vi "运维调试_总磷总氮.vi"() -> ()   [LabVIEW 2016, in "斯坦道总磷总氮.lvlib"]
uses:
  <vilib>/Utility/miscctls.llb/LVPointTypeDef.ctl
  <vilib>/Utility/config.llb/NI_LVConfig.lvlib
  <vilib>/ptbypt/NI_PtbyPt.lvlib
panel:
  in  "总磷参数设置":bool
  in  "总氮参数设置":bool
  in  "模块启用":bool
  in  "串口设置":bool
  in  "备用系数一键写入":bool
  in  "公式一键写入":bool
  in  "流程路径":path=path "C:/Users/std/Documents/斯坦道流程文件/流程.xml"
  in  "曲线模型":cluster{"X^2":dbl, "X":dbl, "B":dbl}(xcontrol)
  out "字符串 2":string
  in  "质控参数设置":bool
  in  "总氮自动测试量程配置":T1
  in  "总磷自动测试量程配置":T1
  out "温度2":sgl
  out "温度1":sgl
  out "ADC":sgl
  out "固件版本号":string
  in  "数组":string[](array[string])
  in  "备用系数写入":bool
  in  "备用系数读取":bool
  in  "备用系数":T2
  in  "量程切换阈值写入":bool
  in  "量程切换阈值读取":bool
  in  "量程切换阈值":cluster{"阈值":dbl, "标液浓度":dbl}
  in  "参数下拉列表":enum16{"总磷", "总氮"}(ring)
  in  "量程下拉列表":enum16{"低量程", "高量程"}(ring)
  in  "测量模式下拉列表":enum16{"水样测量", "零点核查", "跨度核查", "标样核查", "加标回收"}(ring)
  in  "公式":cluster{"X^2":dbl, "X":dbl, "b":dbl}
  in  "写公式":bool
  in  "读公式":bool
  in  "返回":bool
  in  "设置":bool
  out "序列号":string="序列号"
  out "总氮测量数据":T3(xcontrol)
  out "总磷测量数据":T3(xcontrol)
  out "集成报警信息":string
  out "定时启动":bool
  out "总磷总氮运行状态":T4(xcontrol)
  in  "停止":bool
  in  "手动启动":bool
  in  "单步测试":bool
  in  "总磷氨氮调试":u16[](xcontrol)
  out "F3":sgl format="%#.6f"
  out "F2":sgl format="%#.6f"
  out "F1":sgl format="%#.6f"
  out "F0":sgl format="%#.6f"
  out "多列列表框":i32(listbox)
  # "参数设置"
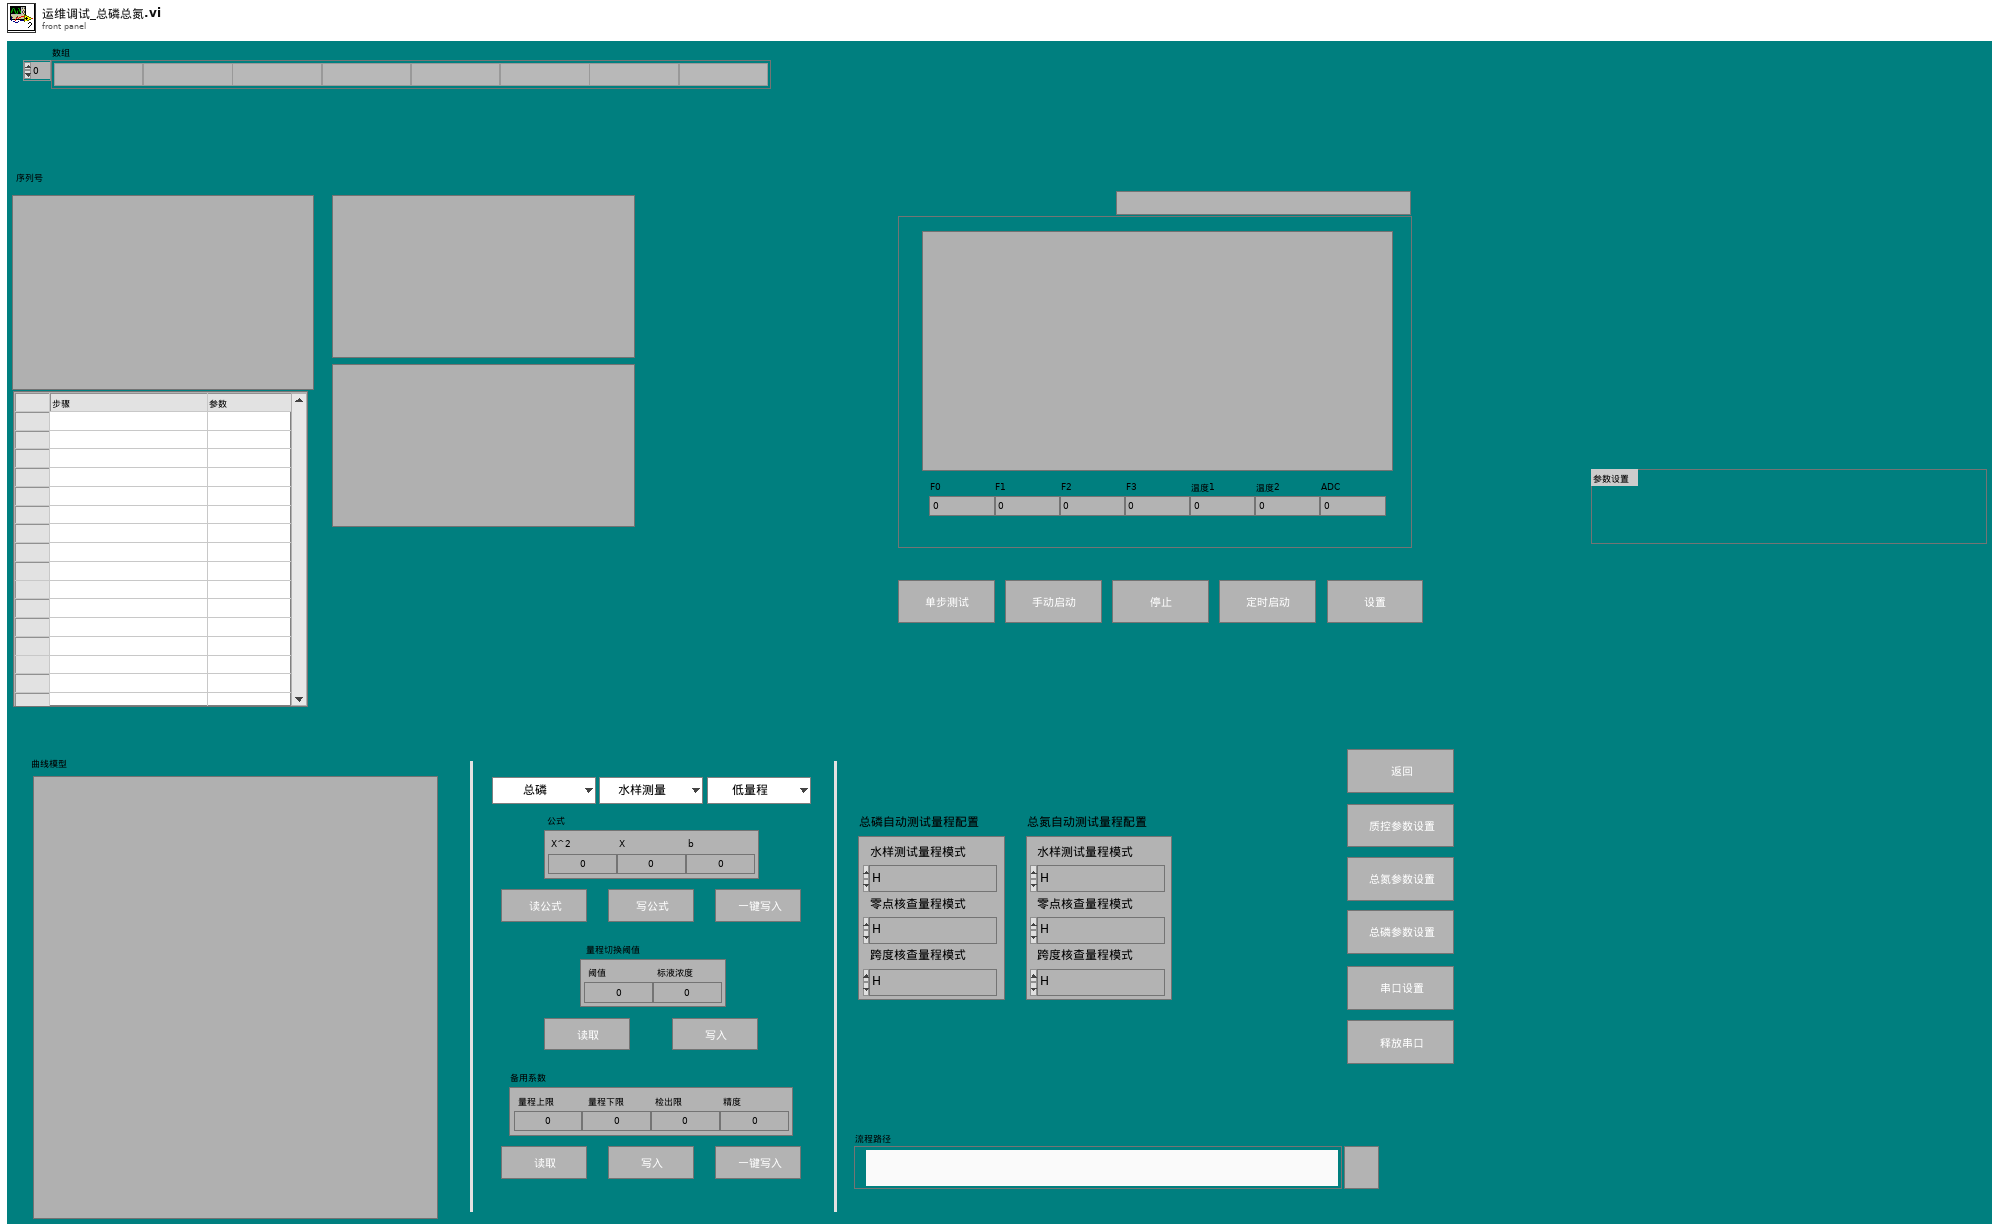
[diagram p1: front panel]
types:
  T1 = cluster{"水样测试量程模式":enum16{"H", "L", "AUTO"}, "空白核查量程模式":enum16{"H", "L", "AUTO"}, "跨度核查量程模式":enum16{"H", "L", "AUTO"}}
  T2 = cluster{"量程上限":dbl, "量程下限":dbl, "检出限":dbl, "精度":dbl}
  T3 = cluster{"flowid":u16, "测量精度":u16, "测量数据区":cluster{"因子编码":u32, "单位":u16, "标样参考值":sgl, "水样数据时间":timestamp, "水样实测值":sgl, "水样数据标识":string, "标样数据时间":timestamp, "标样实测值":sgl, "标样数据标识":string, "空白数据时间":timestamp, "空白实测值":sgl, "空白数据标识":string, "零点核查数据时间":timestamp, "零点核查实测值":sgl, "零点核查数据标识":string, "跨度核查数据时间":timestamp, "跨度核查实测值":sgl, "跨度核查数据标识":string, "加标回收数据时间":timestamp, "加标回收实测值":sgl, "加标回收数据标识":string, "平行样数据时间":timestamp, "平行样实测值":sgl, "平行样数据标识":string, "F0":sgl, "F1":sgl, "F2":sgl, "F3":sgl, "F4":sgl, "F5":sgl, "F6":sgl, "F7":sgl, "温度":sgl, "湿度":sgl, "X值":sgl}}
  T4 = cluster{"系统时间":timestamp, "工作状态":enum16{"空闲", "水样测试", "标样核查", "零点核查", "跨度核查", "空白测试", "平行样测试", "加标回收", "空白校准", "标样校准", "初始化（清洗）"}, "测量模式":enum16{"待机", "连续模式", "周期模式", "定点模式", "受控模式", "手动模式"}, "告警代码":u16, "故障代码":u16, "日志代码":u16, "软件版本":u16, "F0":sgl, "F1":sgl, "F2":sgl, "F3":sgl, "T":sgl, "H":sgl, "id":u16, "flowid":u16, "量程":u16, "总磷控温温度1":sgl, "营养盐控温温度2":sgl, "ADC":sgl}
  T5 = enum16{"启动测量", "标样核查", "零点核查", "跨度核查", "空白测试", "平行样测试", "加标回收", "空白校准", "标样校准", "初始化（清洗）", "停止测试", "仪器重启", "校时", "模式设置", "测量间隔设置"}
  T6 = cluster{"仪器测试类型":enum16{"启动测量", "标样核查", "零点核查", "跨度核查", "空白测试", "平行样测试", "加标回收", "空白校准", "标样校准", "初始化（清洗）", "停止测试", "仪器重启", "校时", "模式设置", "测量间隔设置"}, "周期设置类型":enum16{"定点启动", "间隔启动"}, "定时功能启用":bool, "定时间隔":dbl, "24H周期设置":bool[], "零点核查时间":u16, "跨度核查时间":u16, "质控频次":enum16{"关闭", "每天", "星期一", "星期二", "星期三", "星期四", "星期五", "星期六", "星期日"}}
  T7 = enum16{"关闭", "每天", "星期一", "星期二", "星期三", "星期四", "星期五", "星期六", "星期日"}
  T8 = enum32{"Bad", "Idle", "Run top level", "Running"}
  T9 = typedef "LVDateTimeRec.ctl" = cluster{"秒数的小数部分":dbl, "秒":i32, "分":i32, "时":i32, "日":i32, "月":i32, "年":i32, "天数（周）":i32, "天数（年）":i32, "DST":i32}
  T10 = typedef "LVPointTypeDef.ctl" = cluster{"Horizontal":i16, "Vertical":i16}
  T11 = cluster{"因子编码":u32, "单位":u16, "标样参考值":sgl, "水样数据时间":timestamp, "水样实测值":sgl, "水样数据标识":string, "标样数据时间":timestamp, "标样实测值":sgl, "标样数据标识":string, "空白数据时间":timestamp, "空白实测值":sgl, "空白数据标识":string, "零点核查数据时间":timestamp, "零点核查实测值":sgl, "零点核查数据标识":string, "跨度核查数据时间":timestamp, "跨度核查实测值":sgl, "跨度核查数据标识":string, "加标回收数据时间":timestamp, "加标回收实测值":sgl, "加标回收数据标识":string, "平行样数据时间":timestamp, "平行样实测值":sgl, "平行样数据标识":string, "F0":sgl, "F1":sgl, "F2":sgl, "F3":sgl, "F4":sgl, "F5":sgl, "F6":sgl, "F7":sgl, "温度":sgl, "湿度":sgl, "X值":sgl}
  T12 = enum16{"空闲", "水样测试", "标样核查", "零点核查", "跨度核查", "空白测试", "平行样测试", "加标回收", "空白校准", "标样校准", "初始化（清洗）"}
  T13 = typedef "NI_LVConfig.lvlib/Config Data RefNum.ctl" = refnum<k1>
  T14 = cluster{"启动模式":enum16{"跨度核查", "水样测量", "空白核查", "标样核查", "加标回收"}, "启动参数":u16, "量程":enum16{"低量程", "高量程"}}
  T15 = cluster{"时间标识":timestamp, "设备":string, "日志信息":string, "流程参数":string}
  T16 = cluster{"时间标识":timestamp, "设备":string, "日志信息":string}
  T17 = typedef "LVRowAndColumnUnsignedTypeDef.ctl" = cluster{"Row":u32, "Column":u32}
  T18 = cluster{"参数下拉列表":enum16{"总磷", "总氮"}, "测量模式下拉列表":enum16{"水样测量", "零点核查", "跨度核查", "标样核查", "加标回收"}, "量程下拉列表":enum16{"低量程", "高量程"}}
  T19 = cluster{"站号":u16, "量程切换":enum32{"H", "L", "AUTO"}, "控制命令":enum16{"启动测量", "标样核查", "零点核查", "跨度核查", "空白测试", "平行样测试", "加标回收", "空白校准", "标样校准", "初始化（清洗）", "停止测试", "仪器重启", "校时", "模式设置", "测量间隔设置"}, "模式设置":enum16{"待机", "连续模式", "周期模式", "定点模式", "受控模式", "手动模式"}, "测量间隔":u16}
  T20 = cluster{"总磷跨度值":dbl, "总磷零点标准液浓度":dbl, "总磷跨度标准液浓度":dbl, "总磷标准液标准浓度":dbl, "总氮跨度值":dbl, "总氮零点标准液浓度":dbl, "总氮跨度标准液浓度":dbl, "总氮标准液标准浓度":dbl}
  T21 = cluster{"确定":bool, "总磷跨度值":dbl, "总磷零点标准液浓度":dbl, "总磷跨度标准液浓度":dbl, "总磷标准液标准浓度":dbl, "总氮跨度值":dbl, "总氮零点标准液浓度":dbl, "总氮跨度标准液浓度":dbl, "总氮标准液标准浓度":dbl}
  T22 = cluster{"测量量程":dbl, "测量精度":dbl, "测量间隔":dbl, "消解温度":dbl, "消解时长":dbl, "空白校准时间":timestamp, "曲线截距":dbl, "曲线斜率":dbl, "测量检出限":dbl, "测量信号值":dbl, "线性相关系数":dbl, "二次多项式系数":dbl, "标样校准时间":timestamp, "稀释倍数":dbl, "三项式系数":dbl, "空白标定系数":dbl, "量程系数":dbl, "F0/ORPA":dbl, "F1/ORPB":dbl, "F2/ORPK":dbl, "F3":dbl, "F4":dbl, "F5":dbl, "F6":dbl, "F7":dbl, "X0/滴定数":dbl, "量程":dbl}
  T23 = cluster{"确定":bool, "测量量程":dbl, "测量精度":dbl, "测量间隔":dbl, "消解温度":dbl, "消解时长":dbl, "空白校准时间":timestamp, "曲线截距":dbl, "曲线斜率":dbl, "测量检出限":dbl, "测量信号值":dbl, "线性相关系数":dbl, "二次多项式系数":dbl, "标样校准时间":timestamp, "稀释倍数":dbl, "三项式系数":dbl, "空白标定系数":dbl, "量程系数":dbl, "F0/ORPA":dbl, "F1/ORPB":dbl, "F2/ORPK":dbl, "F3":dbl, "F4":dbl, "F5":dbl, "F6":dbl, "F7":dbl, "X0/滴定数":dbl, "量程":dbl}
  T24 = cluster{"控制命令":enum16{"启动测量", "标样核查", "零点核查", "跨度核查", "空白测试", "平行样测试", "加标回收", "空白校准", "标样校准", "初始化（清洗）", "停止测试", "仪器重启", "校时", "模式设置", "测量间隔设置"}, "周期设置类型":enum16{"定点启动", "间隔启动"}, "定时功能启用":bool, "定时间隔":dbl, "24H周期设置":bool[], "空白核查时间":u16, "跨度核查时间":u16, "质控频次":enum16{"关闭", "每天", "星期一", "星期二", "星期三", "星期四", "星期五", "星期六", "星期日"}}
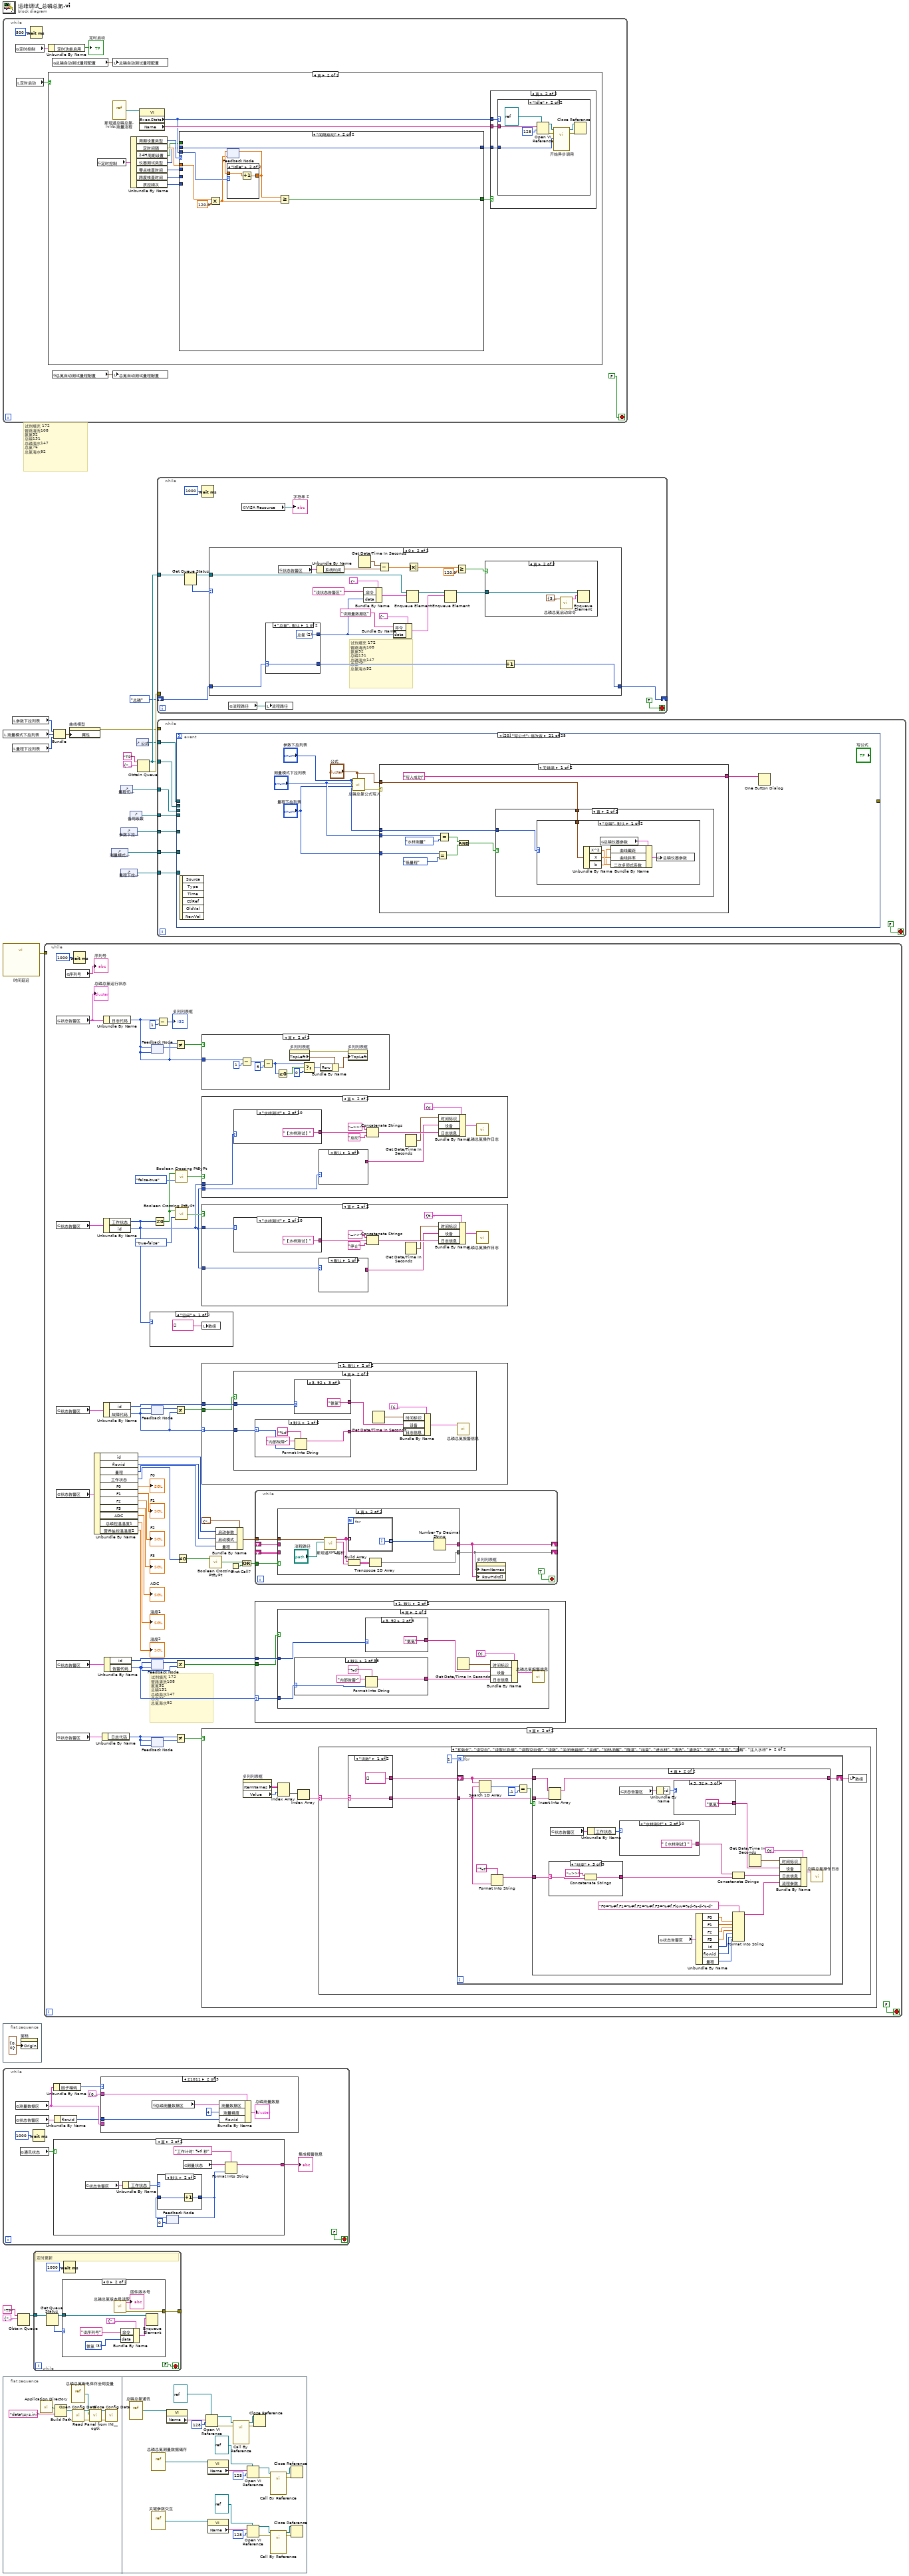
[diagram p0: block diagram]
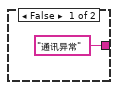
[diagram p3: hidden frame]
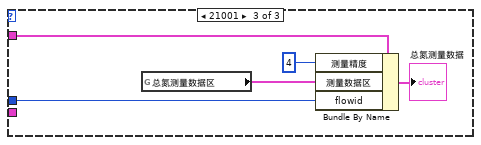
[diagram p6: hidden frame]
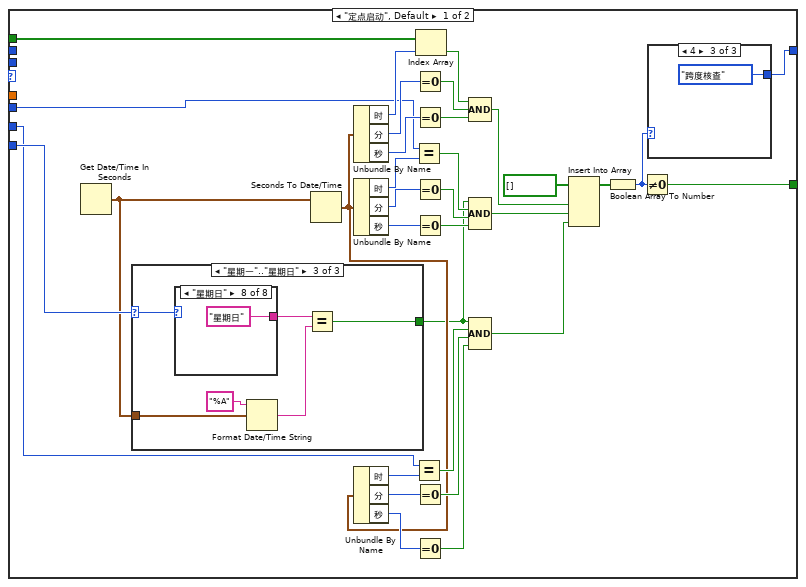
[diagram p8: hidden frame]
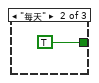
[diagram p10: hidden frame]
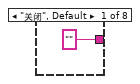
[diagram p11: hidden frame]
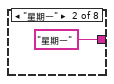
[diagram p12: hidden frame]
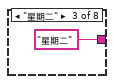
[diagram p13: hidden frame]
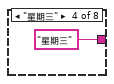
[diagram p14: hidden frame]
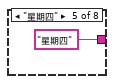
[diagram p15: hidden frame]
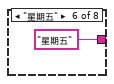
[diagram p16: hidden frame]
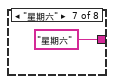
[diagram p17: hidden frame]
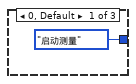
[diagram p18: hidden frame]
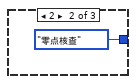
[diagram p19: hidden frame]
diagram:
  # "试剂填充 172 \n管路清洗108\n氨氮92\n总磷131\n总磷海水147\n总氮76\n总氮海水92"
  n1 = while {
    stop <- FALSE stop-if-true
    n2 = global read "总磷总氮断电保存全局变量.vi" "定时控制"() -> (w22:T6)
    n3 = local read "定时启动"() -> (w25:bool)
    n4 = Wait (ms)(milliseconds to wait=u32 500 ("等待时间（毫秒）")) -> ()  [unwired: 1 out]
    n5 = Unbundle By Name(w22) -> ("定时功能启用"=→"定时启动":bool)
    n6 = case shown="真" w25 {
      frame False {
      }
      frame True {
        n7 = global read "总磷总氮断电保存全局变量.vi" "定时控制"() -> (w40:T6)
        n8 = vi-ref "斯坦道总磷总氮.lvlib:测量流程.vi"() -> (w39:refnum<vi>)
        n9 = Unbundle By Name(w40) -> ("周期设置类型"=w37:enum16{"定点启动", "间隔启动"}, "定时间隔"=w35:dbl, "24H周期设置"=w34:bool[], "仪器测试类型"=w33:T5, "零点核查时间"=w32:u16, "跨度核查时间"=w31:u16, "质控频次"=w30:T7)
        n10 = property class="VI"(reference=w39) -> ("Exec.State"=w36:T8, "Name"=w38:string)  [unwired: 1 in, 2 out]
        n11 = case shown="\"间隔启动\"" w37 {
          tunnel: w35 -> [_ w96]
          tunnel: w34 -> [w64 _]
          tunnel: w36 -> [_ w99]
          tunnel: [w42 w94] -> w28
          tunnel: w33 -> [_ w92]
          tunnel: [w68 w92] -> w29
          tunnel: w30 -> [w67 _]
          tunnel: w32 -> [w60 _]
          tunnel: w31 -> [w49 _]
          frame "定点启动", Default {
            n12 = Get Date/Time In Seconds() -> (seconds since 1Jan1904=w66:timestamp)
            n13 = case shown="\"星期一\"..\"星期日\"" w67 {
              selector: w67 -> [_ _ w78]
              tunnel: w66 -> [_ _ w79]
              tunnel: [_ TRUE w75] -> w48
              frame "关闭", Default {
              }
              frame "每天" {
              }
              frame "星期一".."星期日" {
                n14 = case shown="\"星期日\"" w78 {
                  tunnel: ["" ("时间格式字符串(%c)") "星期一" ("时间格式字符串(%c)") "星期二" ("时间格式字符串(%c)") "星期三" ("时间格式字符串(%c)") "星期四" ("时间格式字符串(%c)") "星期五" ("时间格式字符串(%c)") "星期六" ("时间格式字符串(%c)") "星期日" ("时间格式字符串(%c)")] -> w77
                  frame "关闭", Default {
                  }
                  frame "星期一" {
                  }
                  frame "星期二" {
                  }
                  frame "星期三" {
                  }
                  frame "星期四" {
                  }
                  frame "星期五" {
                  }
                  frame "星期六" {
                  }
                  frame "星期日" {
                  }
                }
                n15 = Format Date/Time String(time format string (%c)="%A" ("时间格式字符串(%c)"), seconds (now)=w79) -> (date/time string=w76:string)  [unwired: 1 in]
                n16 = Equal?(x=w77, y=w76) -> (x = y?=w75:bool)
              }
            }
            n17 = Seconds To Date/Time(time stamp (now)=w66) -> (date time rec=w50:T9)  [unwired: 1 in]
            n18 = Unbundle By Name(w50) -> ("时"=w73:i32, "分"=w71:i32, "秒"=w72:i32)
            n19 = Unbundle By Name(w50) -> ("时"=w61:i32, "分"=w63:i32, "秒"=w62:i32)
            n20 = Unbundle By Name(w50) -> ("时"=w53:i32, "分"=w51:i32, "秒"=w52:i32)
            n21 = Equal?(x=w60, y=w61) -> (x = y?=w59:bool)
            n22 = Equal?(x=w49, y=w53) -> (x = y?=w54:bool)
            n23 = Equal To 0?(x=w71) -> (x = 0?=w70:bool)
            n24 = Equal To 0?(x=w72) -> (x = 0?=w69:bool)
            n25 = Equal To 0?(x=w63) -> (x = 0?=w58:bool)
            n26 = Equal To 0?(x=w62) -> (x = 0?=w57:bool)
            n27 = Equal To 0?(x=w51) -> (x = 0?=w55:bool)
            n28 = Equal To 0?(x=w52) -> (x = 0?=w56:bool)
            n29 = Index Array(array=w64, index=w73) -> (element=w65:bool)
            n30 = Compound Arithmetic op=AND ("复合运算")(w65, w70, w69) -> (w46:bool)
            n31 = Compound Arithmetic op=AND ("复合运算")(w48, w59, w58, w57) -> (w45:bool)
            n32 = Compound Arithmetic op=AND ("复合运算")(w48, w54, w55, w56) -> (w44:bool)
            n33 = Insert Into Array(array=bool[] [], new element #1=w46, new element #2=w45, new element #3=w44) -> (w43:bool[])  [unwired: 1 in]
            n34 = Boolean Array To Number(Boolean array=w43) -> (number=w41:u32)
            n35 = Not Equal To 0?(x=w41) -> (x != 0?=w42:bool)
            n36 = case shown="4" w41 {
              tunnel: [T5."启动测量" ("控制命令") T5."零点核查" ("控制命令") T5."跨度核查" ("控制命令")] -> w68
              frame 0, Default {
              }
              frame 2 {
              }
              frame 4 {
              }
            }
          }
          frame "间隔启动" {
            n37 = Multiply(x=w96, y=120.0) -> (x*y=w93:dbl)
            n38 = feedback #1(w93) -> (w98:dbl)
            n39 = case shown="\"Idle\"" w99 {
              tunnel: w98 -> [_ w101]
              tunnel: [_ w100] -> w97
              frame "Bad", Default {
              }
              frame "Idle" {
                n40 = Increment(x=w101) -> (x+1=w100:dbl)
              }
            }
            n41 = feedback-in #1(w97) -> ()
            n42 = Greater Or Equal?(x=w97, y=w93) -> (x >= y?=w94:bool)
          }
        }
        n43 = case shown="真" w28 {
          tunnel: w38 -> [_ w104]
          tunnel: w29 -> [_ w103]
          tunnel: w36 -> [_ w102]
          frame False {
          }
          frame True {
            n44 = case shown="\"Idle\"" w102 {
              tunnel: w104 -> [_ w108]
              tunnel: w103 -> [_ w105]
              frame "Bad", Default {
              }
              frame "Idle" {
                n45 = Open VI Reference(type specifier VI Refnum (for type only)=refnum<vi> refnum, vi path=w108, options=128 ("选项")) -> (vi reference=w109:refnum<vi>, error out=w110:errorcluster)  [unwired: 3 in]
                n46 = call-by-ref "开始异步调用"(reference=w109, error in=w110, "控制命令"=w105) -> (reference out=w111:refnum<vi>, error out=w112:errorcluster)  [unwired: 11 in]
                n47 = Close Reference(reference=w111, error in (no error)=w112) -> ()  [unwired: 1 out]
              }
            }
          }
        }
      }
    }
    n48 = global read "总磷总氮断电保存全局变量.vi" "总磷自动测试量程配置"() -> (w23:T1)
    n49 = global read "总磷总氮断电保存全局变量.vi" "总氮自动测试量程配置"() -> (w24:T1)
    n50 = local write "总磷自动测试量程配置"(w23) -> ()
    n51 = local write "总氮自动测试量程配置"(w24) -> ()
  }
  n52 = local read "测量模式下拉列表"() -> (w3:enum16{"水样测量", "零点核查", "跨度核查", "标样核查", "加标回收"})
  n53 = call "时间延迟"() -> ("error out"=w9:errorcluster)  [unwired: 11 in]
  n54 = flat-sequence {
    frame #0 {
      n55 = property on="窗格" class="Pane"("Origin"=T10 {"Horizontal"=0, "Vertical"=0} ("原点")) -> ()  [unwired: 2 in, 2 out]
    }
  }
  n56 = while {
    stop <- FALSE stop-if-true
    n57 = global read "VAR总磷总氮全局变量.vi" "测量数据区"() -> (w120:T11)
    n58 = global read "VAR总磷总氮全局变量.vi" "状态告警区"() -> (w116:T4)
    n59 = global read "VAR总磷总氮全局变量.vi" "通讯状态"() -> (w118:bool)
    n60 = Wait (ms)(milliseconds to wait=u32 1000 ("等待时间（毫秒）")) -> ()  [unwired: 1 out]
    n61 = Unbundle By Name(w120) -> ("因子编码"=w119:u32)
    n62 = case shown="真" w118 {
      tunnel: ["通讯异常" ("集成报警信息") w125] -> w117
      frame False {
      }
      frame True {
        n63 = global read "VAR总磷总氮全局变量.vi" "状态告警区"() -> (w131:T4)
        n64 = Unbundle By Name(w131) -> ("工作状态"=w130:T12)
        n65 = feedback #2(0) -> (w128:i32)
        n66 = case shown="默认" w130 {
          tunnel: w128 -> [_ w133]
          tunnel: [_ w132] -> w126
          frame "空闲" {
          }
          frame Default {
            n67 = Increment(x=w133) -> (x+1=w132:i32)
          }
        }
        n68 = feedback-in #2(w126) -> ()
        n69 = global read "VAR总磷总氮全局变量.vi" "测量状态"() -> (w124:string)
        n70 = Format Into String(format string="工作计时: %d 秒" ("格式字符串"), initial string=w124, w126) -> (resulting string=w125:string)  [unwired: 1 in, 1 out]
      }
    }
    "集成报警信息" <- w117
    n71 = Unbundle By Name(w116) -> ("flowid"=w115:u16)
    n72 = case shown="21011" w119 {
      tunnel: w120 -> [_ _ _]
      tunnel: w115 -> [_ w136 w142]
      tunnel: T3 {"flowid"=0, "测量精度"=0, "测量数据区"={"因子编码"=0, "单位"=0, "标样参考值"=0.0, "水样数据时间"=timestamp(0 s since 1904-01-01), "水样实测值"=0.0, "水样数据标识"="", "标样数据时间"=timestamp(0 s since 1904-01-01), "标样实测值"=0.0, "标样数据标识"="", "空白数据时间"=timestamp(0 s since 1904-01-01), "空白实测值"=0.0, "空白数据标识"="", "零点核查数据时间"=timestamp(0 s since 1904-01-01), "零点核查实测值"=0.0, "零点核查数据标识"="", "跨度核查数据时间"=timestamp(0 s since 1904-01-01), "跨度核查实测值"=0.0, "跨度核查数据标识"="", "加标回收数据时间"=timestamp(0 s since 1904-01-01), "加标回收实测值"=0.0, "加标回收数据标识"="", "平行样数据时间"=timestamp(0 s since 1904-01-01), "平行样实测值"=0.0, "平行样数据标识"="", "F0"=0.0, "F1"=0.0, "F2"=0.0, "F3"=0.0, "F4"=0.0, "F5"=0.0, "F6"=0.0, "F7"=0.0, "温度"=0.0, "湿度"=0.0, "X值"=0.0}} ("总氮测量数据") -> [_ w135 w141]
      frame Default {
      }
      frame 21011 {
        n73 = global read "VAR总磷总氮全局变量.vi" "总磷测量数据区"() -> (w134:T11)
        n74 = Bundle By Name(cluster=w135, "测量数据区"=w134, "测量精度"=u16 4, "flowid"=w136) -> (→"总磷测量数据":T3)
      }
      frame 21001 {
        n75 = global read "VAR总磷总氮全局变量.vi" "总氮测量数据区"() -> (w139:T11)
        n76 = Bundle By Name(cluster=w141, "测量精度"=u16 4, "测量数据区"=w139, "flowid"=w142) -> (→"总氮测量数据":T3)
      }
    }
  }
  n77 = flat-sequence {
    frame #0 {
      n78 = call <vilib>:"Application Directory.vi"() -> ("Application Directory"=w151:path)
      n79 = Build Path(base path=w151, name or relative path="data\\sys.ini" ("名称或相对路径")) -> (appended path=w149:path)
      n80 = vi-ref "总磷总氮断电保存全局变量.vi"() -> (w147:refnum<vi>)
      n81 = call <vilib>:"Open Config Data.vi"("configuration file path"=w149) -> ("error out"=w145:errorcluster, "refnum"=w148:T13)  [unwired: 8 in, 1 out]
      n82 = call <userlib>:"Read Panel from INI__ogtk.vi"("error in (no error)"=w145, "VI ref"=w147, "refnum"=w148) -> ("error out"=w144:errorcluster, "refnum out"=w146:T13)  [unwired: 7 in]
      n83 = call <vilib>:"Close Config Data.vi"("error in (no error)"=w144, "refnum"=w146) -> ()  [unwired: 8 in, 2 out]
    }
    frame #1 {
      n84 = vi-ref "总磷总氮通讯.vi"() -> (w175:refnum<vi>)
      n85 = vi-ref "总磷总氮测量数据储存.vi"() -> (w167:refnum<vi>)
      n86 = vi-ref "关键参数交互.vi"() -> (w152:refnum<vi>)
      n87 = property class="VI"(reference=w175) -> ("Name"=w174:string)  [unwired: 1 in, 2 out]
      n88 = Open VI Reference(type specifier VI Refnum (for type only)=refnum<vi> refnum, vi path=w174, options=128 ("选项")) -> (vi reference=w172:refnum<vi>, error out=w170:errorcluster)  [unwired: 3 in]
      n89 = property class="VI"(reference=w167) -> ("Name"=w160:string)  [unwired: 1 in, 2 out]
      n90 = property class="VI"(reference=w152) -> ("Name"=w159:string)  [unwired: 1 in, 2 out]
      n91 = call-by-ref "?"(reference=w172, error in=w170) -> (reference out=w168:refnum<vi>, error out=w169:errorcluster)  [unwired: 12 in]
      n92 = Open VI Reference(type specifier VI Refnum (for type only)=refnum<vi> refnum, vi path=w160, options=128 ("选项")) -> (vi reference=w162:refnum<vi>, error out=w164:errorcluster)  [unwired: 3 in]
      n93 = Open VI Reference(type specifier VI Refnum (for type only)=refnum<vi> refnum, vi path=w159, options=128 ("选项")) -> (vi reference=w157:refnum<vi>, error out=w155:errorcluster)  [unwired: 3 in]
      n94 = Close Reference(reference=w168, error in (no error)=w169) -> ()  [unwired: 1 out]
      n95 = call-by-ref "?"(reference=w162, error in=w164) -> (reference out=w166:refnum<vi>, error out=w165:errorcluster)  [unwired: 12 in]
      n96 = call-by-ref "?"(reference=w157, error in=w155) -> (reference out=w153:refnum<vi>, error out=w154:errorcluster)  [unwired: 12 in]
      n97 = Close Reference(reference=w166, error in (no error)=w165) -> ()  [unwired: 1 out]
      n98 = Close Reference(reference=w153, error in (no error)=w154) -> ()  [unwired: 1 out]
    }
  }
  n99 = local read "参数下拉列表"() -> (w2:enum16{"总磷", "总氮"})
  n100 = local read "量程下拉列表"() -> (w1:enum16{"低量程", "高量程"})
  n101 = Obtain Queue(name (unnamed)="TP" ("名称（未命名）"), element data type=cluster{"命令":string, "data":variant} {"命令"="", "data"=variant}) -> (queue out=w6:refnum<queue>)  [unwired: 3 in, 2 out]
  n102 = while {
    tunnel: w6 -> [w180]
    tunnel: [w178] -> _
    stop <- FALSE stop-if-true
    # "定时更新"
    n103 = Get Queue Status(queue=w180) -> (queue out=w177:refnum<queue>, # elements in queue=w176:i32)  [unwired: 2 in, 6 out]
    n104 = case shown="0" w176 {
      tunnel: w177 -> [_ w185]
      tunnel: [_ w182] -> w178
      frame Default {
      }
      frame 0 {
        w186 = u16 3 items=["总磷"=1, "氨氮"=3] ("站号")
        n105 = call "总磷总氮版本号读取.vi"() -> ("error out"=w182:errorcluster, "固件版本号"=→"固件版本号":string)  [unwired: 10 in]
        n106 = Bundle By Name(cluster=cluster{"命令":string, "data":variant} {"命令"="", "data"=variant} ("元素"), "命令"="读序列号", "data"=w186) -> (w184:cluster{"命令":string, "data":variant})
        n107 = Enqueue Element(queue=w185, element=w184) -> ()  [unwired: 2 in, 3 out]
      }
    }
    n108 = Wait (ms)(milliseconds to wait=u32 1000 ("等待时间（毫秒）")) -> ()  [unwired: 1 out]
  }
  n109 = while {
    tunnel: w9 -> [_]
    stop <- FALSE stop-if-true
    # "试剂填充 172 \n管路清洗108\n氨氮92\n总磷131\n总磷海水147\n总氮76\n总氮海水92"
    n110 = global read "VAR总磷总氮全局变量.vi" "状态告警区"() -> (w222:T4)
    "总磷总氮运行状态" <- w222
    n111 = global read "VAR总磷总氮全局变量.vi" "状态告警区"() -> (w209:T4)
    n112 = global read "VAR总磷总氮全局变量.vi" "状态告警区"() -> (w214:T4)
    n113 = global read "VAR总磷总氮全局变量.vi" "状态告警区"() -> (w230:T4)
    n114 = global read "VAR总磷总氮全局变量.vi" "状态告警区"() -> (w219:T4)
    n115 = global read "VAR总磷总氮全局变量.vi" "状态告警区"() -> (w207:T4)
    n116 = global read "VAR总磷总氮全局变量.vi" "序列号"() -> (→"序列号":string)
    n117 = Wait (ms)(milliseconds to wait=u32 1000 ("等待时间（毫秒）")) -> ()  [unwired: 1 out]
    n118 = Unbundle By Name(w230) -> ("id"=w227:u16, "flowid"=w229:u16, "量程"=w228:u16, "工作状态"=w197:T12, "F0"=→"F0":sgl, "F1"=→"F1":sgl, "F2"=→"F2":sgl, "F3"=→"F3":sgl, "ADC"=→"ADC":sgl, "总磷控温温度1"=→"温度1":sgl, "营养盐控温温度2"=→"温度2":sgl)
    n119 = Unbundle By Name(w207) -> ("日志代码"=w206:u16)
    n120 = Unbundle By Name(w222) -> ("日志代码"=w203:u16)
    n121 = Unbundle By Name(w209) -> ("工作状态"=w190:T12, "id"=w189:u16)
    n122 = Unbundle By Name(w214) -> ("id"=w213:u16, "故障代码"=w210:u16)
    n123 = Unbundle By Name(w219) -> ("id"=w218:u16, "告警代码"=w215:u16)
    n124 = case shown="\"空闲\"" w190 {
      frame "空闲" {
        n125 = local write "数组"(string[] [] ("数组")) -> ()
      }
      frame "水样测试", Default {
      }
    }
    n126 = feedback-in #3(w203) -> ()
    n127 = feedback #3(w203) -> (w235:u16)
    n128 = feedback #4(w210) -> (w211:u16)
    n129 = feedback-in #4(w210) -> ()
    n130 = feedback #5(w215) -> (w216:u16)
    n131 = feedback-in #5(w215) -> ()
    n132 = feedback #6(w206) -> (w208:u16)
    n133 = feedback-in #6(w206) -> ()
    n134 = Not Equal To 0?(x=w190) -> (x != 0?=w192:bool)
    n135 = Subtract(x=w203, y=1) -> (x-y=→"多列列表框":i32)
    n136 = Not Equal?(x=w203, y=w235) -> (x != y?=w234:bool)
    n137 = Not Equal?(x=w211, y=w210) -> (x != y?=w212:bool)
    n138 = Not Equal?(x=w216, y=w215) -> (x != y?=w217:bool)
    n139 = Not Equal?(x=w206, y=w208) -> (x != y?=w205:bool)
    n140 = call <vilib>:"Boolean Crossing PtByPt.vi"("direction"=enum16{"either", "false-true", "true-false"}."false-true", "input"=w192) -> ("crossing"=w194:bool)  [unwired: 1 in]
    n141 = call <vilib>:"Boolean Crossing PtByPt.vi"("direction"=enum16{"either", "false-true", "true-false"}."true-false", "input"=w192) -> ("crossing"=w191:bool)  [unwired: 1 in]
    n142 = Not Equal To 0?(x=w197) -> (x != 0?=w232:bool)
    n143 = case shown="真" w234 {
      tunnel: w203 -> [_ w445]
      frame False {
      }
      frame True {
        n144 = Subtract(x=w445, y=1) -> (x-y=w443:i32)
        n145 = Subtract(x=w443, y=5) -> (x-y=w447:i32)
        n146 = Greater Or Equal To 0?(x=w447) -> (x >= 0?=w446:bool)
        n147 = property on="多列列表框" class="MCListbox (严格)"() -> (error out=w451:errorcluster, "TopLeft"=w452:T17)  [unwired: 2 in, 1 out]
        n148 = Select(t=w447, s=w446, f=0) -> (s? t:f=w448:i32)
        n149 = Bundle By Name(cluster=w452, "Row"=w448) -> (w453:T17)
        n150 = property on="多列列表框" class="MCListbox (严格)"(error in=w451, "TopLeft"=w453) -> ()  [unwired: 1 in, 2 out]
      }
    }
    n151 = case shown="真" w194 {
      tunnel: w190 -> [_ w262]
      tunnel: w189 -> [_ w261]
      frame False {
      }
      frame True {
        n152 = case shown="\"水样测试\"" w262 {
          tunnel: [_ "【水样测试】" ("字符串") "【标样核查】" ("字符串") "【零点核查】" ("字符串") "【跨度核查】" ("字符串") "【空白测试】" ("字符串") "【平行样测试】" ("字符串") "【加标回收】" ("字符串") "【空白校准】" ("字符串") "【标样校准】" ("字符串")] -> w269
          frame "空闲", Default {
          }
          frame "水样测试" {
          }
          frame "标样核查" {
          }
          frame "零点核查" {
          }
          frame "跨度核查" {
          }
          frame "空白测试" {
          }
          frame "平行样测试" {
          }
          frame "加标回收" {
          }
          frame "空白校准" {
          }
          frame "标样校准" {
          }
        }
        n153 = case shown="默认" w261 {
          tunnel: [_ "总磷" ("table输入") "氨氮" ("table输入") "总氮" ("table输入")] -> w265
          frame Default {
          }
          frame 1, 131 {
          }
          frame 3, 92 {
          }
          frame 2, 76 {
          }
        }
        n154 = Concatenate Strings("-->>" ("字符串"), w269, "启动" ("字符串")) -> (w268:string)
        n155 = Get Date/Time In Seconds() -> (seconds since 1Jan1904=w266:timestamp)
        n156 = Bundle By Name(cluster=T15 {"时间标识"=timestamp(0 s since 1904-01-01), "设备"="", "日志信息"="", "流程参数"=""} ("data in"), "时间标识"=w266, "设备"=w265, "日志信息"=w268) -> (w260:T15)
        n157 = call "总磷总氮操作日志.vi"("data in"=w260) -> ()  [unwired: 11 in]
      }
    }
    n158 = case shown="真" w191 {
      tunnel: w190 -> [_ w240]
      tunnel: w189 -> [_ w239]
      frame False {
      }
      frame True {
        n159 = case shown="\"水样测试\"" w240 {
          tunnel: [_ "【水样测试】" ("字符串") "【标样核查】" ("字符串") "【零点核查】" ("字符串") "【跨度核查】" ("字符串") "【空白测试】" ("字符串") "【平行样测试】" ("字符串") "【加标回收】" ("字符串") "【空白校准】" ("字符串") "【标样校准】" ("字符串")] -> w247
          frame "空闲", Default {
          }
          frame "水样测试" {
          }
          frame "标样核查" {
          }
          frame "零点核查" {
          }
          frame "跨度核查" {
          }
          frame "空白测试" {
          }
          frame "平行样测试" {
          }
          frame "加标回收" {
          }
          frame "空白校准" {
          }
          frame "标样校准" {
          }
        }
        n160 = case shown="默认" w239 {
          tunnel: [_ "总磷" ("table输入") "氨氮" ("table输入") "总氮" ("table输入")] -> w243
          frame Default {
          }
          frame 1, 131 {
          }
          frame 3, 92 {
          }
          frame 2, 76 {
          }
        }
        n161 = Concatenate Strings("-->>" ("字符串"), w247, "停止" ("字符串")) -> (w246:string)
        n162 = Get Date/Time In Seconds() -> (seconds since 1Jan1904=w244:timestamp)
        n163 = Bundle By Name(cluster=T15 {"时间标识"=timestamp(0 s since 1904-01-01), "设备"="", "日志信息"="", "流程参数"=""} ("data in"), "时间标识"=w244, "设备"=w243, "日志信息"=w246) -> (w238:T15)
        n164 = call "总磷总氮操作日志.vi"("data in"=w238) -> ()  [unwired: 11 in]
      }
    }
    n165 = case shown="1, 默认" w210 {
      selector: w210 -> [_ w350]
      tunnel: w213 -> [_ w351]
      tunnel: w212 -> [_ w349]
      frame 0 {
      }
      frame 1, Default {
        n166 = case shown="真" w349 {
          tunnel: w351 -> [_ w358]
          tunnel: w350 -> [_ w353]
          frame False {
          }
          frame True {
            n167 = case shown="默认" w353 {
              selector: w353 -> [w360 _ _ _ _ _]
              tunnel: [w359 "无故障" "电机故障" "温度故障" "通讯故障" "滴定故障"] -> w352
              frame Default {
                n168 = Format Into String(format string="%d" ("格式字符串"), initial string="内部故障-" ("工作状态"), w360) -> (resulting string=w359:string)  [unwired: 1 in, 1 out]
              }
              frame 0 {
              }
              frame 1 {
              }
              frame 2 {
              }
              frame 3 {
              }
              frame 4 {
              }
            }
            n169 = case shown="3, 92" w358 {
              tunnel: [_ "总磷" ("table输入") "氨氮" ("table输入") "总氮" ("table输入")] -> w354
              frame Default {
              }
              frame 1, 131 {
              }
              frame 3, 92 {
              }
              frame 2, 76 {
              }
            }
            n170 = Get Date/Time In Seconds() -> (seconds since 1Jan1904=w355:timestamp)
            n171 = Bundle By Name(cluster=T16 {"时间标识"=timestamp(0 s since 1904-01-01), "设备"="", "日志信息"=""} ("data in"), "时间标识"=w355, "设备"=w354, "日志信息"=w352) -> (w356:T16)
            n172 = call "总磷总氮报警信息.vi"("data in"=w356) -> ()  [unwired: 10 in, 1 out]
          }
        }
      }
    }
    n173 = case shown="真" w205 {
      frame False {
      }
      frame True {
        n174 = property on="多列列表框" class="MCListbox (严格)"() -> ("ItemNames"=w285:string[][], "Value"=w286:i32)  [unwired: 2 in, 2 out]
        n175 = Index Array(array=w285, index (row)=w286) -> (element=w284:string[])  [unwired: 1 in]
        n176 = Index Array(array=w284) -> (element=w283:string)  [unwired: 1 in]
        n177 = case shown="\"初始化\", \"读空白\", \"读取比色值\", \"读取空白值\", \"读数\", \"关闭电磁阀\", \"关阀\", \"加热消解\", \"降温\", \"结束\", \"进水样\", \"清洗\", \"清洗1\", \"润洗\", \"显色\", \"消解\", \"注入水样\"" w283 {
          selector: w283 -> [_ w289]
          frame Default {
          }
          frame "初始化", "读空白", "读取比色值", "读取空白值", "读数", "关闭电磁阀", "关阀", "加热消解", "降温", "结束", "进水样", "清洗", "清洗1", "润洗", "显色", "消解", "注入水样" {
            n178 = case shown="\"读数\"" w289 {
              selector: w289 -> [w293 w295]
              tunnel: [w293 w295] -> w288
              tunnel: [string[] [] ("数组") "数组"] -> w287
              frame "读数" {
              }
              frame Default {
              }
            }
            n179 = for {
              N: 1 -> [_]
              tunnel: w288 -> [w297]
              shift-right: [w296] -> w290
              shift-left: w287 -> [w298]
              n180 = Search 1D Array(1D array=w298, element=w297) -> (index of element=w301:i32)  [unwired: 1 in]
              n181 = Format Into String(format string="%s" ("格式字符串"), w297) -> (resulting string=w302:string)  [unwired: 2 in, 1 out]
              n182 = Equal?(x=w301, y=-1) -> (x = y?=w299:bool)
              n183 = case shown="真" w299 {
                tunnel: w302 -> [_ w310]
                tunnel: w298 -> [w304 w314]
                tunnel: w297 -> [_ w313]
                tunnel: [w304 w312] -> w296
                frame False {
                }
                frame True {
                  n184 = Insert Into Array(array=w314, new element=w313) -> (w312:string[])  [unwired: 1 in]
                  n185 = case shown="\"结束\"" w310 {
                    selector: w310 -> [w339 w342 w345]
                    tunnel: [w339 w341 w344] -> w309
                    frame Default {
                    }
                    frame "初始化" {
                      n186 = Concatenate Strings("-->>" ("字符串"), w342) -> (w341:string)
                    }
                    frame "结束" {
                      n187 = Concatenate Strings("-->>" ("字符串"), w345) -> (w344:string)
                    }
                  }
                  n188 = global read "VAR总磷总氮全局变量.vi" "状态告警区"() -> (w308:T4)
                  n189 = Unbundle By Name(w308) -> ("工作状态"=w307:T12)
                  n190 = global read "VAR总磷总氮全局变量.vi" "状态告警区"() -> (w329:T4)
                  n191 = case shown="\"水样测试\"" w307 {
                    tunnel: [_ "【水样测试】" ("字符串") "【标样核查】" ("字符串") "【零点核查】" ("字符串") "【跨度核查】" ("字符串") "【空白测试】" ("字符串") "【平行样测试】" ("字符串") "【加标回收】" ("字符串") "【空白校准】" ("字符串") "【标样校准】" ("字符串")] -> w305
                    frame "空闲", Default {
                    }
                    frame "水样测试" {
                    }
                    frame "标样核查" {
                    }
                    frame "零点核查" {
                    }
                    frame "跨度核查" {
                    }
                    frame "空白测试" {
                    }
                    frame "平行样测试" {
                    }
                    frame "加标回收" {
                    }
                    frame "空白校准" {
                    }
                    frame "标样校准" {
                    }
                  }
                  n192 = Unbundle By Name(w329) -> ("id"=w328:u16)
                  n193 = global read "VAR总磷总氮全局变量.vi" "状态告警区"() -> (w324:T4)
                  n194 = case shown="3, 92" w328 {
                    tunnel: [_ "总磷" ("table输入") "氨氮" ("table输入") "总氮" ("table输入")] -> w326
                    frame Default {
                    }
                    frame 1, 131 {
                    }
                    frame 3, 92 {
                    }
                    frame 2, 76 {
                    }
                  }
                  n195 = Unbundle By Name(w324) -> ("F0"=w321:sgl, "F1"=w320:sgl, "F2"=w319:sgl, "F3"=w318:sgl, "id"=w317:u16, "flowid"=w316:u16, "量程"=w315:u16)
                  n196 = Concatenate Strings(w305, w309) -> (w306:string)
                  n197 = Format Into String(format string="F0=%#f,F1=%#f,F2=%#f,F3=%#f,Flow=%d-%-d-%-d" ("格式字符串"), w321, w320, w319, w318, w317, w316, w315) -> (resulting string=w322:string)  [unwired: 2 in, 1 out]
                  n198 = Get Date/Time In Seconds() -> (seconds since 1Jan1904=w325:timestamp)
                  n199 = Bundle By Name(cluster=T15 {"时间标识"=timestamp(0 s since 1904-01-01), "设备"="", "日志信息"="", "流程参数"=""} ("data in"), "时间标识"=w325, "设备"=w326, "日志信息"=w306, "流程参数"=w322) -> (w327:T15)
                  n200 = call "总磷总氮操作日志.vi"("data in"=w327) -> ()  [unwired: 11 in]
                }
              }
            }
            n201 = local write "数组"(w290) -> ()
          }
        }
      }
    }
    n202 = call <vilib>:"Boolean Crossing PtByPt.vi"("input"=w232) -> ("crossing"=w196:bool)  [unwired: 2 in]
    n203 = Bundle By Name(cluster=T14 {"启动模式"=enum."跨度核查", "启动参数"=1, "量程"=enum."低量程"} ("参数簇"), "启动参数"=w227, "启动模式"=w229, "量程"=w228) -> (w221:T14)
    n204 = First Call?() -> (First Call?: T/F=w233:bool)
    n205 = Or(x=w196, y=w233) -> (x .or. y?=w231:bool)
    n206 = while {
      tunnel: w231 -> [w431]
      tunnel: w221 -> [w430]
      shift-right: [w425] -> _
      shift-left: _ -> [w427]
      shift-right: [w426] -> _
      shift-left: _ -> [w428]
      stop <- TRUE stop-if-true
      n207 = case shown="真" w431 {
        tunnel: [w433 w441] -> w426
        tunnel: [w432 w440] -> w425
        tunnel: w430 -> [_ w435]
        tunnel: w428 -> [w433 _]
        tunnel: w427 -> [w432 _]
        frame False {
        }
        frame True {
          n208 = call "斯坦道XML解析.vi"("添加的路径"="流程路径", "参数簇"=w435) -> ("步骤时间"=w436:string[], "步骤名"=w438:string[])  [unwired: 8 in]
          n209 = for {
            tunnel: w438 -> [_] mode=indexing
            tunnel: [w442] -> w439 mode=indexing
            i -> [w442]
          }
          n210 = Build Array(w438, w436) -> (w437:string[][])
          n211 = Transpose 2D Array(2D array=w437) -> (transposed array=w440:string[][])
          n212 = Number To Decimal String(number=w439) -> (decimal integer string=w441:string[])  [unwired: 1 in]
        }
      }
      n213 = property on="多列列表框" class="MCListbox (严格)"("ItemNames"=w425, "RowHdrs[]"=w426) -> ()  [unwired: 2 in, 2 out]
    }
    n214 = case shown="1, 默认" w215 {
      selector: w215 -> [_ w372]
      tunnel: w218 -> [_ w373]
      tunnel: w217 -> [_ w371]
      frame 0 {
      }
      frame 1, Default {
        n215 = case shown="真" w371 {
          tunnel: w373 -> [_ w380]
          tunnel: w372 -> [_ w374]
          frame False {
          }
          frame True {
            n216 = case shown="默认" w374 {
              selector: w374 -> [w382 _ _ _ _ _ _ _ _ _ _ _ _ _ _ _ _ _ _ _ _ _ _ _ _ _ _ _ _ _ _ _ _ _ _ _ _ _]
              tunnel: [w381 "无告警" "缺试剂告警" "缺水样告警" "缺蒸馏水告警" "缺标液告警" "仪表漏液告警" "标定异常告警" "超量程告警" "加热异常" "低试剂预警" "超上限告警" "超下限告警" "仪表内部其他异常" "滴定异常告警" "电极异常告警" "量程切换告警" "参数设置告警" "PH电极电位异常" "电导率电极异常" "浊度光度异常" "溶解氧电极异常" "溶解氧光强异常" "温度异常告警" "PH异常告警" "溶解氧异常告警" "电导率异常告警" "浊度异常告警" "叶绿素异常告警" "藻密度异常告警" "蓝绿藻异常告警" "ORP异常告警" "氨氮异常告警" "清洁刷异常告警" "SD卡异常告警" "蓝牙异常告警" "WiFi异常告警" "流程异常告警"] -> w375
              frame Default {
                n217 = Format Into String(format string="%d" ("格式字符串"), initial string="内部告警-" ("工作状态"), w382) -> (resulting string=w381:string)  [unwired: 1 in, 1 out]
              }
              frame 0 {
              }
              frame 1 {
              }
              frame 2 {
              }
              frame 3 {
              }
              frame 4 {
              }
              frame 5 {
              }
              frame 6 {
              }
              frame 7 {
              }
              frame 8 {
              }
              frame 9 {
              }
              frame 10 {
              }
              frame 11 {
              }
              frame 12 {
              }
              frame 13 {
              }
              frame 14 {
              }
              frame 15 {
              }
              frame 16 {
              }
              frame 17 {
              }
              frame 18 {
              }
              frame 19 {
              }
              frame 20 {
              }
              frame 21 {
              }
              frame 22 {
              }
              frame 23 {
              }
              frame 24 {
              }
              frame 25 {
              }
              frame 26 {
              }
              frame 27 {
              }
              frame 28 {
              }
              frame 29 {
              }
              frame 30 {
              }
              frame 31 {
              }
              frame 32 {
              }
              frame 33 {
              }
              frame 34 {
              }
              frame 35 {
              }
              frame 36 {
              }
            }
            n218 = case shown="3, 92" w380 {
              tunnel: ["总磷" ("table输入") "氨氮" ("table输入") "总氮" ("table输入")] -> w376
              frame 1, 131 {
              }
              frame 3, 92 {
              }
              frame 2, 76, Default {
              }
            }
            n219 = Get Date/Time In Seconds() -> (seconds since 1Jan1904=w377:timestamp)
            n220 = Bundle By Name(cluster=T16 {"时间标识"=timestamp(0 s since 1904-01-01), "设备"="", "日志信息"=""} ("data in"), "时间标识"=w377, "设备"=w376, "日志信息"=w375) -> (w378:T16)
            n221 = call "总磷总氮报警信息.vi"("data in"=w378) -> ()  [unwired: 10 in, 1 out]
          }
        }
      }
    }
  }
  n222 = Bundle("参数下拉列表"=w2, "测量模式下拉列表"=w3, "量程下拉列表"=w1) -> (w4:T18)  [unwired: 1 in]
  n223 = property on="曲线模型" class="曲线模型 (严格)"("属性"=w4) -> (error out=w5:errorcluster)  [unwired: 2 in, 1 out]
  n224 = control-ref of="测量模式下拉列表"() -> (w13:refnum<vi>)
  n225 = control-ref of="量程切换阈值"() -> (w11:refnum<vi>)
  n226 = control-ref of="参数下拉列表"() -> (w14:refnum<vi>)
  n227 = control-ref of="量程下拉列表"() -> (w15:refnum<vi>)
  n228 = control-ref of="备用系数"() -> (w10:refnum<vi>)
  n229 = control-ref of="公式"() -> (w12:refnum<vi>)
  n230 = Obtain Queue(name (unnamed)="TP" ("名称（未命名）"), element data type=cluster{"命令":string, "data":variant} {"命令"="", "data"=variant}) -> (queue out=w17:refnum<queue>, error out=w18:errorcluster)  [unwired: 3 in, 1 out]
  n231 = while {
    tunnel: w17 -> [w460]
    tunnel: w18 -> [_]
    shift-right: [w458] -> _
    shift-left: enum16{"总磷", "总氮"}."总磷" ("枚举") -> [w459]
    stop <- FALSE stop-if-true
    n232 = Get Queue Status(queue=w460) -> (queue out=w455:refnum<queue>, # elements in queue=w454:i32)  [unwired: 2 in, 6 out]
    n233 = Wait (ms)(milliseconds to wait=u32 1000 ("等待时间（毫秒）")) -> ()  [unwired: 1 out]
    n234 = case shown="0" w454 {
      tunnel: w459 -> [w463 w483]
      tunnel: [w463 w482] -> w458
      tunnel: w455 -> [_ w481]
      frame Default {
      }
      frame 0 {
        # "试剂填充 172 \n管路清洗108\n氨氮92\n总磷131\n总磷海水147\n总氮76\n总氮海水92"
        n235 = case shown="\"总氮\", 默认" w483 {
          selector: w483 -> [w487 w489]
          tunnel: [w488 w490] -> w473
          tunnel: [w487 w489] -> w472
          frame "总氮", Default {
            w488 = u16 2 items=["总磷"=1, "总氮"=2] ("站号")
          }
          frame "总磷" {
            w490 = u16 1 items=["总磷"=1, "氨氮"=3] ("站号")
          }
        }
        n236 = global read "VAR总磷总氮全局变量.vi" "状态告警区"() -> (w464:T4)
        n237 = Unbundle By Name(w464) -> ("系统时间"=w471:timestamp)
        n238 = Get Date/Time In Seconds() -> (seconds since 1Jan1904=w470:timestamp)
        n239 = Bundle By Name(cluster=cluster{"命令":string, "data":variant} {"命令"="", "data"=variant} ("元素"), "命令"="读状态告警区", "data"=w473) -> (w479:cluster{"命令":string, "data":variant})
        n240 = Subtract(x=w470, y=w471) -> (x-y=w469:dbl)
        n241 = Bundle By Name(cluster=cluster{"命令":string, "data":variant} {"命令"="", "data"=variant} ("元素"), "命令"="读测量数据区", "data"=w473) -> (w476:cluster{"命令":string, "data":variant})
        n242 = Enqueue Element(queue=w481, element=w479) -> (queue out=w474:refnum<queue>)  [unwired: 2 in, 2 out]
        n243 = Absolute Value(x=w469) -> (abs(x)=w468:dbl)
        n244 = Enqueue Element(queue=w474, element=w476) -> (queue out=w465:refnum<queue>)  [unwired: 2 in, 2 out]
        n245 = Greater Or Equal?(x=w468, y=120.0) -> (x >= y?=w466:bool)
        n246 = case shown="真" w466 {
          tunnel: w465 -> [_ w485]
          frame False {
          }
          frame True {
            n247 = call "总磷总氮启动命令.vi"("参数"=T19 {"站号"=3, "量程切换"=enum."AUTO", "控制命令"=enum."校时", "模式设置"=enum."待机", "测量间隔"=0}) -> ("启动命令"=w484:cluster{"命令":string, "data":variant})  [unwired: 10 in]
            n248 = Enqueue Element(queue=w485, element=w484) -> ()  [unwired: 2 in, 3 out]
          }
        }
        n249 = Increment(x=w472) -> (x+1=w482:enum16{"总磷", "总氮"})
      }
    }
    n250 = global read "总磷总氮断电保存全局变量.vi" "流程路径"() -> (w457:path)
    n251 = global read "总磷总氮断电保存全局变量.vi" "VISA Resource"() -> (→"字符串 2":refnum<visa-resource-name>)
    n252 = local write "流程路径"(w457) -> ()
  }
  n253 = while {
    tunnel: w17 -> [w497]
    tunnel: w15 -> [w496]
    tunnel: w14 -> [w495]
    tunnel: w13 -> [w494]
    tunnel: w12 -> [w493]
    tunnel: w11 -> [w492]
    tunnel: w10 -> [w491]
    tunnel: w5 -> [_]
    stop <- FALSE stop-if-true
    n254 = event shown="[20] \"写公式\": 值改变" {
      selector: _ -> [_ _ _ _ _ _ _ _ _ _ _ _ _ _ _ _ _ _ _ _ _ _ _ _ _]
      dyn-events: _ -> [_ _ _ _ _ _ _ _ _ _ _ _ _ _ _ _ _ _ _ _ _ _ _ _ _]
      timeout: _ -> [_ _ _ _ _ _ _ _ _ _ _ _ _ _ _ _ _ _ _ _ _ _ _ _ _]
      tunnel: w497 -> [_ _ w513 w541 _ _ _ _ _ _ _ _ w683 _ w708 w712 _ _ _ _ _ _ _ _ _]
      tunnel: w496 -> [_ _ _ _ _ _ _ _ _ _ _ _ _ _ _ _ _ _ _ w728 _ w771 w780 w788 w799]
      tunnel: w495 -> [_ _ _ _ _ _ _ _ _ _ _ _ _ _ _ _ _ _ _ w726 _ w769 w782 w794 w805]
      tunnel: w494 -> [_ _ _ _ _ _ _ _ _ _ _ _ _ _ _ _ _ _ _ w727 _ w770 w781 w787 w800]
      tunnel: w493 -> [_ _ _ _ _ _ _ _ _ _ _ _ _ _ _ _ _ _ _ w722 _ _ _ _ _]
      tunnel: w492 -> [_ _ _ _ _ _ _ _ _ _ _ _ _ _ _ _ _ _ _ _ _ w765 _ _ _]
      tunnel: w491 -> [_ _ _ _ _ _ _ _ _ _ _ _ _ _ _ _ _ _ _ _ _ _ _ w792 _]
      tunnel: [_ w499 _ _ _ _ _ _ _ _ _ _ _ _ _ _ _ _ _ _ _ _ _ _ _] -> _
      event Timeout {
        n255 = event-data() -> ()  [unwired: 1 in, 3 out]
      }
      event "测量模式下拉列表", "量程下拉列表", "参数下拉列表": Value Change {
        n256 = event-data() -> ()  [unwired: 1 in, 6 out]
        n257 = local read "测量模式下拉列表"() -> (w501:enum16{"水样测量", "零点核查", "跨度核查", "标样核查", "加标回收"})
        n258 = local read "参数下拉列表"() -> (w502:enum16{"总磷", "总氮"})
        n259 = local read "量程下拉列表"() -> (w503:enum16{"低量程", "高量程"})
        n260 = Bundle("参数下拉列表"=w502, "测量模式下拉列表"=w501, "量程下拉列表"=w503) -> (w500:T18)  [unwired: 1 in]
        n261 = property on="曲线模型" class="曲线模型 (严格)"("属性"=w500) -> (error out=w499:errorcluster)  [unwired: 2 in, 1 out]
      }
      event "串口设置": Value Change {
        n262 = event-data() -> ()  [unwired: 1 in, 6 out]
        n263 = global read "总磷总氮断电保存全局变量.vi" "MB通信方式选择"() -> (w504:enum16{"串口", "TCP"})
        n264 = global read "总磷总氮断电保存全局变量.vi" "VISA Resource"() -> (w510:refnum<visa-resource-name>)
        n265 = global read "总磷总氮断电保存全局变量.vi" "PORT"() -> (w508:string)
        n266 = global read "总磷总氮断电保存全局变量.vi" "IP"() -> (w509:string)
        n267 = call "串口配置.vi"("PORT"=w508, "IP"=w509, "MB通信方式选择"=w504, "请选择串口:"=w510) -> ("PORT 2"=w506:string, "IP 2"=w507:string, "确认 2"=w511:bool, "VISA资源名称 2"=w512:refnum<visa-resource-name>, "MB通信方式选择 2"=w505:enum16{"串口", "TCP"})  [unwired: 3 in]
        n268 = case shown="真" w511 {
          tunnel: w512 -> [_ w518]
          tunnel: w513 -> [_ w517]
          tunnel: w507 -> [_ w516]
          tunnel: w506 -> [_ w515]
          tunnel: w505 -> [_ w514]
          frame False {
          }
          frame True {
            n269 = flat-sequence {
              tunnel: w518 -> [w523]
              tunnel: w517 -> [w524]
              tunnel: w516 -> [w522]
              tunnel: w515 -> [w521]
              tunnel: w514 -> [w520]
              frame #0 {
                n270 = global write "总磷总氮断电保存全局变量.vi" "IP"(w522) -> ()
                n271 = global write "总磷总氮断电保存全局变量.vi" "PORT"(w521) -> ()
                n272 = global write "总磷总氮断电保存全局变量.vi" "VISA Resource"(w523) -> ()
                n273 = global write "总磷总氮断电保存全局变量.vi" "MB通信方式选择"(w520) -> ()
                n274 = Flush Queue(queue=w524) -> (queue out=w519:refnum<queue>)  [unwired: 1 in, 2 out]
                n275 = Enqueue Element(queue=w519, element=cluster{"命令":string, "data":variant} {"命令"="启用模块", "data"=variant} ("元素")) -> ()  [unwired: 2 in, 3 out]
              }
              frame #1 {
                n276 = call <vilib>:"Application Directory.vi"() -> ("Application Directory"=w539:path)
                n277 = Build Path(base path=w539, name or relative path="data\\sys.ini" ("名称或相对路径")) -> (appended path=w537:path)
                n278 = call <vilib>:"Open Config Data.vi"("configuration file path"=w537) -> ("error out"=w533:errorcluster, "refnum"=w536:T13)  [unwired: 8 in, 1 out]
                n279 = vi-ref "斯坦道总磷总氮.lvlib:总磷总氮断电保存全局变量.vi"() -> (w535:refnum<vi>)
                n280 = call <userlib>:"Write Panel to INI__ogtk.vi"("error in (no error)"=w533, "VI ref"=w535, "refnum"=w536) -> ("error out"=w532:errorcluster, "refnum out"=w534:T13)  [unwired: 7 in]
                n281 = call <vilib>:"Close Config Data.vi"("error in (no error)"=w532, "refnum"=w534) -> ("error out"=w527:errorcluster, "file path"=w526:path)  [unwired: 8 in]
                n282 = Open/Create/Replace File(file path (use dialog)=w526, error in=w527) -> (refnum out=w530:refnum<file>, error out=w531:errorcluster)  [unwired: 4 in, 1 out]
                n283 = Flush File(refnum=w530, error in=w531) -> (refnum out=w529:refnum<file>, error out=w528:errorcluster)
                n284 = Close File(refnum=w529, error in=w528) -> ()  [unwired: 2 out]
              }
            }
          }
        }
      }
      event "模块启用": Value Change {
        n285 = event-data() -> ("OldVal"=w542:bool)  [unwired: 1 in, 5 out]
        n286 = Flush Queue(queue=w541) -> (queue out=w540:refnum<queue>)  [unwired: 1 in, 2 out]
        n287 = case shown="假" w542 {
          tunnel: w540 -> [w543 w545]
          frame False {
            n288 = Enqueue Element(queue=w543, element=cluster{"命令":string, "data":variant} {"命令"="停用模块", "data"=variant} ("元素")) -> ()  [unwired: 2 in, 3 out]
          }
          frame True {
            n289 = Enqueue Element(queue=w545, element=cluster{"命令":string, "data":variant} {"命令"="启用模块", "data"=variant} ("元素")) -> ()  [unwired: 2 in, 3 out]
          }
        }
      }
      event "流程路径": Value Change {
        n290 = event-data() -> ()  [unwired: 1 in, 6 out]
        n291 = flat-sequence {
          frame #0 {
            n292 = local read "流程路径"() -> (w547:path)
            n293 = global write "总磷总氮断电保存全局变量.vi" "流程路径"(w547) -> ()
          }
          frame #1 {
            n294 = call <vilib>:"Application Directory.vi"() -> ("Application Directory"=w561:path)
            n295 = Build Path(base path=w561, name or relative path="data\\sys.ini" ("名称或相对路径")) -> (appended path=w559:path)
            n296 = call <vilib>:"Open Config Data.vi"("configuration file path"=w559) -> ("error out"=w555:errorcluster, "refnum"=w558:T13)  [unwired: 8 in, 1 out]
            n297 = vi-ref "总磷总氮断电保存全局变量.vi"() -> (w557:refnum<vi>)
            n298 = call <userlib>:"Write Panel to INI__ogtk.vi"("error in (no error)"=w555, "VI ref"=w557, "refnum"=w558) -> ("error out"=w554:errorcluster, "refnum out"=w556:T13)  [unwired: 7 in]
            n299 = call <vilib>:"Close Config Data.vi"("error in (no error)"=w554, "refnum"=w556) -> ("error out"=w549:errorcluster, "file path"=w548:path)  [unwired: 8 in]
            n300 = Open/Create/Replace File(file path (use dialog)=w548, error in=w549) -> (refnum out=w552:refnum<file>, error out=w553:errorcluster)  [unwired: 4 in, 1 out]
            n301 = Flush File(refnum=w552, error in=w553) -> (refnum out=w551:refnum<file>, error out=w550:errorcluster)
            n302 = Close File(refnum=w551, error in=w550) -> ()  [unwired: 2 out]
          }
        }
      }
      event "公式一键写入": Value Change {
        n303 = event-data() -> ()  [unwired: 1 in, 6 out]
        n304 = local read "公式"() -> (w562:cluster{"X^2":dbl, "X":dbl, "b":dbl})
        n305 = call "公式复合写入.vi"("公式"=w562) -> ()  [unwired: 11 in]
      }
      event "备用系数一键写入": Value Change {
        n306 = event-data() -> ()  [unwired: 1 in, 6 out]
        n307 = local read "备用系数"() -> (w563:T2)
        n308 = call "量程参数复合参数写入.vi"("备用系数"=w563) -> ()  [unwired: 11 in]
      }
      event "曲线模型": Value Change {
        n309 = event-data() -> ()  [unwired: 1 in, 6 out]
        n310 = local write "公式"("曲线模型") -> ()
      }
      event "质控参数设置": Value Change {
        n311 = event-data() -> ()  [unwired: 1 in, 6 out]
        n312 = global read "总磷总氮断电保存全局变量.vi" "质控参数设置"() -> (w565:T20)
        n313 = call "总磷总氮质控参数设置.vi"("质控参数设置"=w565) -> ("输出簇"=w566:T21)  [unwired: 10 in]
        n314 = Unbundle By Name(w566) -> ("确定"=w567:bool)
        n315 = case shown="真" w567 {
          tunnel: w566 -> [_ w569]
          tunnel: w565 -> [_ w568]
          frame False {
          }
          frame True {
            n316 = flat-sequence {
              tunnel: w569 -> [w580]
              tunnel: w568 -> [w579]
              frame #0 {
                n317 = Unbundle By Name(w580) -> ("总磷跨度值"=w578:dbl, "总磷零点标准液浓度"=w577:dbl, "总磷跨度标准液浓度"=w576:dbl, "总磷标准液标准浓度"=w575:dbl, "总氮跨度值"=w574:dbl, "总氮零点标准液浓度"=w573:dbl, "总氮跨度标准液浓度"=w572:dbl, "总氮标准液标准浓度"=w571:dbl)
                n318 = Bundle By Name(cluster=w579, "总磷跨度值"=w578, "总磷零点标准液浓度"=w577, "总磷跨度标准液浓度"=w576, "总磷标准液标准浓度"=w575, "总氮跨度值"=w574, "总氮零点标准液浓度"=w573, "总氮跨度标准液浓度"=w572, "总氮标准液标准浓度"=w571) -> (w570:T20)
                n319 = global write "总磷总氮断电保存全局变量.vi" "质控参数设置"(w570) -> ()
              }
              frame #1 {
                n320 = call <vilib>:"Application Directory.vi"() -> ("Application Directory"=w594:path)
                n321 = Build Path(base path=w594, name or relative path="data\\sys.ini" ("名称或相对路径")) -> (appended path=w592:path)
                n322 = call <vilib>:"Open Config Data.vi"("configuration file path"=w592) -> ("error out"=w588:errorcluster, "refnum"=w591:T13)  [unwired: 8 in, 1 out]
                n323 = vi-ref "总磷总氮断电保存全局变量.vi"() -> (w590:refnum<vi>)
                n324 = call <userlib>:"Write Panel to INI__ogtk.vi"("error in (no error)"=w588, "VI ref"=w590, "refnum"=w591) -> ("error out"=w587:errorcluster, "refnum out"=w589:T13)  [unwired: 7 in]
                n325 = call <vilib>:"Close Config Data.vi"("error in (no error)"=w587, "refnum"=w589) -> ("error out"=w582:errorcluster, "file path"=w581:path)  [unwired: 8 in]
                n326 = Open/Create/Replace File(file path (use dialog)=w581, error in=w582) -> (refnum out=w585:refnum<file>, error out=w586:errorcluster)  [unwired: 4 in, 1 out]
                n327 = Flush File(refnum=w585, error in=w586) -> (refnum out=w584:refnum<file>, error out=w583:errorcluster)
                n328 = Close File(refnum=w584, error in=w583) -> ()  [unwired: 2 out]
              }
            }
          }
        }
      }
      event "总氮参数设置": Value Change {
        n329 = event-data() -> ()  [unwired: 1 in, 6 out]
        n330 = global read "总磷总氮断电保存全局变量.vi" "总氮仪器参数"() -> (w596:T22)
        n331 = call "仪器参数设置.vi"("氨氮仪器参数"=w596) -> ("仪器参数设置输出"=w595:T23)  [unwired: 10 in]
        n332 = Unbundle By Name(w595) -> ("确定"=w597:bool)
        n333 = case shown="真" w597 {
          tunnel: w595 -> [_ w599]
          tunnel: w596 -> [_ w598]
          frame False {
          }
          frame True {
            n334 = flat-sequence {
              tunnel: w599 -> [w615]
              tunnel: w598 -> [w614]
              frame #0 {
                n335 = Unbundle By Name(w615) -> ("测量量程"=w613:dbl, "测量精度"=w612:dbl, "测量间隔"=w611:dbl, "消解温度"=w610:dbl, "消解时长"=w609:dbl, "空白校准时间"=w608:timestamp, "曲线截距"=w607:dbl, "曲线斜率"=w606:dbl, "测量检出限"=w604:dbl, "测量信号值"=w603:dbl, "线性相关系数"=w602:dbl, "二次多项式系数"=w601:dbl, "标样校准时间"=w600:timestamp)
                n336 = Bundle By Name(cluster=w614, "测量量程"=w613, "测量精度"=w612, "测量间隔"=w611, "消解温度"=w610, "消解时长"=w609, "空白校准时间"=w608, "曲线截距"=w607, "曲线斜率"=w606, "测量检出限"=w604, "测量信号值"=w603, "线性相关系数"=w602, "二次多项式系数"=w601, "标样校准时间"=w600) -> (w605:T22)
                n337 = global write "总磷总氮断电保存全局变量.vi" "总氮仪器参数"(w605) -> ()
              }
              frame #1 {
                n338 = call <vilib>:"Application Directory.vi"() -> ("Application Directory"=w629:path)
                n339 = Build Path(base path=w629, name or relative path="data\\sys.ini" ("名称或相对路径")) -> (appended path=w627:path)
                n340 = call <vilib>:"Open Config Data.vi"("configuration file path"=w627) -> ("error out"=w623:errorcluster, "refnum"=w626:T13)  [unwired: 8 in, 1 out]
                n341 = vi-ref "总磷总氮断电保存全局变量.vi"() -> (w625:refnum<vi>)
                n342 = call <userlib>:"Write Panel to INI__ogtk.vi"("error in (no error)"=w623, "VI ref"=w625, "refnum"=w626) -> ("error out"=w622:errorcluster, "refnum out"=w624:T13)  [unwired: 7 in]
                n343 = call <vilib>:"Close Config Data.vi"("error in (no error)"=w622, "refnum"=w624) -> ("error out"=w617:errorcluster, "file path"=w616:path)  [unwired: 8 in]
                n344 = Open/Create/Replace File(file path (use dialog)=w616, error in=w617) -> (refnum out=w620:refnum<file>, error out=w621:errorcluster)  [unwired: 4 in, 1 out]
                n345 = Flush File(refnum=w620, error in=w621) -> (refnum out=w619:refnum<file>, error out=w618:errorcluster)
                n346 = Close File(refnum=w619, error in=w618) -> ()  [unwired: 2 out]
              }
            }
          }
        }
      }
      event "总磷参数设置": Value Change {
        n347 = event-data() -> ()  [unwired: 1 in, 6 out]
        n348 = global read "总磷总氮断电保存全局变量.vi" "总磷仪器参数"() -> (w631:T22)
        n349 = call "仪器参数设置.vi"("氨氮仪器参数"=w631) -> ("仪器参数设置输出"=w630:T23)  [unwired: 10 in]
        n350 = Unbundle By Name(w630) -> ("确定"=w632:bool)
        n351 = case shown="真" w632 {
          tunnel: w630 -> [_ w634]
          tunnel: w631 -> [_ w633]
          frame False {
          }
          frame True {
            n352 = flat-sequence {
              tunnel: w634 -> [w650]
              tunnel: w633 -> [w649]
              frame #0 {
                n353 = Unbundle By Name(w650) -> ("测量量程"=w648:dbl, "测量精度"=w647:dbl, "测量间隔"=w646:dbl, "消解温度"=w645:dbl, "消解时长"=w644:dbl, "空白校准时间"=w643:timestamp, "曲线截距"=w642:dbl, "曲线斜率"=w641:dbl, "测量检出限"=w639:dbl, "测量信号值"=w638:dbl, "线性相关系数"=w637:dbl, "二次多项式系数"=w636:dbl, "标样校准时间"=w635:timestamp)
                n354 = Bundle By Name(cluster=w649, "测量量程"=w648, "测量精度"=w647, "测量间隔"=w646, "消解温度"=w645, "消解时长"=w644, "空白校准时间"=w643, "曲线截距"=w642, "曲线斜率"=w641, "测量检出限"=w639, "测量信号值"=w638, "线性相关系数"=w637, "二次多项式系数"=w636, "标样校准时间"=w635) -> (w640:T22)
                n355 = global write "总磷总氮断电保存全局变量.vi" "总磷仪器参数"(w640) -> ()
              }
              frame #1 {
                n356 = call <vilib>:"Application Directory.vi"() -> ("Application Directory"=w664:path)
                n357 = Build Path(base path=w664, name or relative path="data\\sys.ini" ("名称或相对路径")) -> (appended path=w662:path)
                n358 = call <vilib>:"Open Config Data.vi"("configuration file path"=w662) -> ("error out"=w658:errorcluster, "refnum"=w661:T13)  [unwired: 8 in, 1 out]
                n359 = vi-ref "总磷总氮断电保存全局变量.vi"() -> (w660:refnum<vi>)
                n360 = call <userlib>:"Write Panel to INI__ogtk.vi"("error in (no error)"=w658, "VI ref"=w660, "refnum"=w661) -> ("error out"=w657:errorcluster, "refnum out"=w659:T13)  [unwired: 7 in]
                n361 = call <vilib>:"Close Config Data.vi"("error in (no error)"=w657, "refnum"=w659) -> ("error out"=w652:errorcluster, "file path"=w651:path)  [unwired: 8 in]
                n362 = Open/Create/Replace File(file path (use dialog)=w651, error in=w652) -> (refnum out=w655:refnum<file>, error out=w656:errorcluster)  [unwired: 4 in, 1 out]
                n363 = Flush File(refnum=w655, error in=w656) -> (refnum out=w654:refnum<file>, error out=w653:errorcluster)
                n364 = Close File(refnum=w654, error in=w653) -> ()  [unwired: 2 out]
              }
            }
          }
        }
      }
      event "总磷自动测试量程配置", "总氮自动测试量程配置": Value Change {
        n365 = event-data() -> ()  [unwired: 1 in, 6 out]
        n366 = flat-sequence {
          frame #0 {
            n367 = global write "总磷总氮断电保存全局变量.vi" "总氮自动测试量程配置"("总氮自动测试量程配置") -> ()
            n368 = global write "总磷总氮断电保存全局变量.vi" "总磷自动测试量程配置"("总磷自动测试量程配置") -> ()
          }
          frame #1 {
            n369 = call <vilib>:"Application Directory.vi"() -> ("Application Directory"=w680:path)
            n370 = Build Path(base path=w680, name or relative path="data\\sys.ini" ("名称或相对路径")) -> (appended path=w678:path)
            n371 = call <vilib>:"Open Config Data.vi"("configuration file path"=w678) -> ("error out"=w674:errorcluster, "refnum"=w677:T13)  [unwired: 8 in, 1 out]
            n372 = vi-ref "总磷总氮断电保存全局变量.vi"() -> (w676:refnum<vi>)
            n373 = call <userlib>:"Write Panel to INI__ogtk.vi"("error in (no error)"=w674, "VI ref"=w676, "refnum"=w677) -> ("error out"=w673:errorcluster, "refnum out"=w675:T13)  [unwired: 7 in]
            n374 = call <vilib>:"Close Config Data.vi"("error in (no error)"=w673, "refnum"=w675) -> ("error out"=w668:errorcluster, "file path"=w667:path)  [unwired: 8 in]
            n375 = Open/Create/Replace File(file path (use dialog)=w667, error in=w668) -> (refnum out=w671:refnum<file>, error out=w672:errorcluster)  [unwired: 4 in, 1 out]
            n376 = Flush File(refnum=w671, error in=w672) -> (refnum out=w670:refnum<file>, error out=w669:errorcluster)
            n377 = Close File(refnum=w670, error in=w669) -> ()  [unwired: 2 out]
          }
        }
      }
      event "手动启动": Value Change {
        n378 = event-data() -> ()  [unwired: 1 in, 6 out]
        n379 = call "总磷总氮启动参数对话框.vi"() -> ("确认"=w681:bool, "元素"=w682:cluster{"命令":string, "data":variant})  [unwired: 10 in]
        n380 = case shown="真" w681 {
          tunnel: w683 -> [_ w685]
          tunnel: w682 -> [_ w684]
          frame False {
          }
          frame True {
            n381 = Enqueue Element(queue=w685, element=w684) -> ()  [unwired: 2 in, 3 out]
          }
        }
      }
      event "定时启动": Mouse Down {
        n382 = event-data() -> ()  [unwired: 1 in, 6 out]
        n383 = flat-sequence {
          frame #0 {
            n384 = global read "总磷总氮断电保存全局变量.vi" "定时控制"() -> (w687:T6)
            n385 = call "总磷总氮周期设置.vi"("定时控制输入"=w687) -> ("定时控制输出"=w686:T24)  [unwired: 10 in]
            n386 = global write "总磷总氮断电保存全局变量.vi" "定时控制"(w686) -> ()
          }
          frame #1 {
            n387 = call <vilib>:"Application Directory.vi"() -> ("Application Directory"=w701:path)
            n388 = Build Path(base path=w701, name or relative path="data\\sys.ini" ("名称或相对路径")) -> (appended path=w699:path)
            n389 = call <vilib>:"Open Config Data.vi"("configuration file path"=w699) -> ("error out"=w695:errorcluster, "refnum"=w698:T13)  [unwired: 8 in, 1 out]
            n390 = vi-ref "总磷总氮断电保存全局变量.vi"() -> (w697:refnum<vi>)
            n391 = call <userlib>:"Write Panel to INI__ogtk.vi"("error in (no error)"=w695, "VI ref"=w697, "refnum"=w698) -> ("error out"=w694:errorcluster, "refnum out"=w696:T13)  [unwired: 7 in]
            n392 = call <vilib>:"Close Config Data.vi"("error in (no error)"=w694, "refnum"=w696) -> ("error out"=w689:errorcluster, "file path"=w688:path)  [unwired: 8 in]
            n393 = Open/Create/Replace File(file path (use dialog)=w688, error in=w689) -> (refnum out=w692:refnum<file>, error out=w693:errorcluster)  [unwired: 4 in, 1 out]
            n394 = Flush File(refnum=w692, error in=w693) -> (refnum out=w691:refnum<file>, error out=w690:errorcluster)
            n395 = Close File(refnum=w691, error in=w690) -> ()  [unwired: 2 out]
          }
        }
      }
      event "单步测试": Value Change {
        w703 = u16 1 items=["总磷"=1, "氨氮"=3] ("站号")
        n396 = event-data() -> ()  [unwired: 1 in, 6 out]
        n397 = Bundle("站号"=w703, "总磷氨氮调试"="总磷氨氮调试") -> (w702:cluster{"站号":u16, "总磷氨氮调试":u16[]})  [unwired: 1 in]
        n398 = Bundle By Name(cluster=cluster{"命令":string, "data":variant} {"命令"="", "data"=variant} ("元素"), "命令"="debug", "data"=w702) -> (w705:cluster{"命令":string, "data":variant})
        n399 = Enqueue Element(queue=w708, element=w705) -> ()  [unwired: 2 in, 3 out]
      }
      event "停止": Value Change {
        n400 = event-data() -> ()  [unwired: 1 in, 6 out]
        n401 = Enqueue Element(queue=w712, element=cluster{"命令":string, "data":variant} {"命令"="启动", "data"=variant(cluster{"站号":u16, "控制命令输出":u16[]} {"站号"=1, "控制命令输出"=[2816]})} ("元素")) -> (queue out=w709:refnum<queue>)  [unwired: 2 in, 2 out]
        n402 = Enqueue Element(queue=w709, element=cluster{"命令":string, "data":variant} {"命令"="启动", "data"=variant(cluster{"站号":u16, "控制命令输出":u16[]} {"站号"=2, "控制命令输出"=[2816]})} ("元素")) -> ()  [unwired: 2 in, 3 out]
      }
      event "设置": Value Change {
        n403 = event-data() -> ()  [unwired: 1 in, 6 out]
        n404 = property on="窗格" class="Pane"("Origin"=T10 {"Horizontal"=0, "Vertical"=628} ("原点")) -> ()  [unwired: 2 in, 2 out]
      }
      event "返回": Value Change {
        n405 = event-data() -> ()  [unwired: 1 in, 6 out]
        n406 = property on="窗格" class="Pane"("Origin"=T10 {"Horizontal"=0, "Vertical"=0} ("原点")) -> ()  [unwired: 2 in, 2 out]
      }
      event "公式.X^2", "公式.X", "公式.b", "量程切换阈值.阈值", "量程切换阈值.标液浓度", "备用系数.量程上限", "备用系数.量程下限", "备用系数.检出限", "备用系数.精度": Mouse Down {
        n407 = event-data() -> ("CtlRef"=w718:refnum<vi>)  [unwired: 1 in, 5 out]
        n408 = property class="DigNum (严格)"(reference=w718) -> (reference out=w716:refnum<vi>, "Value"=w717:dbl)  [unwired: 1 in, 1 out]
        n409 = call "数字键盘.vi"("OldNumber"=w717) -> ("NewNumber"=w715:dbl)
        n410 = property class="DigNum (严格)"(reference=w716, "Val(Sgnl)"=w715) -> ()  [unwired: 1 in, 2 out]
      }
      event "读公式": Value Change {
        n411 = event-data() -> ()  [unwired: 1 in, 6 out]
        n412 = property class="Enum (严格)"(reference=w726) -> ("Value"=w725:enum16{"总磷", "总氮"})  [unwired: 1 in, 2 out]
        n413 = property class="Enum (严格)"(reference=w727) -> ("Value"=w724:enum16{"水样测量", "零点核查", "跨度核查", "标样核查", "加标回收"})  [unwired: 1 in, 2 out]
        n414 = property class="Enum (严格)"(reference=w728) -> ("Value"=w723:enum16{"低量程", "高量程"})  [unwired: 1 in, 2 out]
        n415 = call "总磷总氮公式读取.vi"("量程"=w723, "测量模式"=w724, "测量参数"=w725) -> ("error out"=w720:errorcluster, "公式"=w721:cluster{"X^2":dbl, "X":dbl, "b":dbl})  [unwired: 7 in]
        n416 = property class="Clust (严格)"(reference=w722, "Value"=w721) -> ()  [unwired: 1 in, 2 out]
        n417 = case shown="错误" w720 {
          tunnel: ["读取成功" ("消息") "读取失败" ("消息")] -> w719
          frame No Error {
          }
          frame Error {
          }
        }
        n418 = One Button Dialog(message=w719) -> ()  [unwired: 1 in, 1 out]
      }
      event "写公式": Value Change {
        n419 = event-data() -> ()  [unwired: 1 in, 6 out]
        n420 = call "总磷总氮公式写入.vi"("公式"="公式", "量程"="量程下拉列表", "测量模式"="测量模式下拉列表", "测量参数"="参数下拉列表") -> ("error out"=w735:errorcluster)  [unwired: 7 in]
        n421 = case shown="无错误" w735 {
          tunnel: ["写入成功" ("消息") "写入失败" ("消息")] -> w736
          tunnel: "公式" -> [w745 _]
          tunnel: "测量模式下拉列表" -> [w743 _]
          tunnel: "量程下拉列表" -> [w741 _]
          tunnel: "参数下拉列表" -> [w740 _]
          frame No Error {
            n422 = Equal?(x=w741, y=enum16{"低量程", "高量程"}."低量程" ("量程下拉列表")) -> (x = y?=w738:bool)
            n423 = Equal?(x=w743, y=enum16{"水样测量", "零点核查", "跨度核查", "标样核查", "加标回收"}."水样测量" ("测量模式下拉列表")) -> (x = y?=w739:bool)
            n424 = And(x=w739, y=w738) -> (x .and. y?=w737:bool)
            n425 = case shown="真" w737 {
              tunnel: w745 -> [_ w748]
              tunnel: w740 -> [_ w747]
              frame False {
              }
              frame True {
                n426 = case shown="\"总磷\", 默认" w747 {
                  tunnel: w748 -> [w749 w755]
                  frame "总磷", Default {
                    n427 = Unbundle By Name(w749) -> ("X^2"=w752:dbl, "X"=w751:dbl, "b"=w750:dbl)
                    n428 = global read "总磷总氮断电保存全局变量.vi" "总磷仪器参数"() -> (w753:T22)
                    n429 = Bundle By Name(cluster=w753, "曲线截距"=w750, "曲线斜率"=w751, "二次多项式系数"=w752) -> (w754:T22)
                    n430 = global write "总磷总氮断电保存全局变量.vi" "总磷仪器参数"(w754) -> ()
                  }
                  frame "总氮" {
                    n431 = Unbundle By Name(w755) -> ("X^2"=w758:dbl, "X"=w757:dbl, "b"=w756:dbl)
                    n432 = global read "总磷总氮断电保存全局变量.vi" "总氮仪器参数"() -> (w759:T22)
                    n433 = Bundle By Name(cluster=w759, "曲线截距"=w756, "曲线斜率"=w757, "二次多项式系数"=w758) -> (w760:T22)
                    n434 = global write "总磷总氮断电保存全局变量.vi" "总氮仪器参数"(w760) -> ()
                  }
                }
              }
            }
          }
          frame Error {
          }
        }
        n435 = One Button Dialog(message=w736) -> ()  [unwired: 1 in, 1 out]
      }
      event "量程切换阈值读取": Value Change {
        n436 = event-data() -> ()  [unwired: 1 in, 6 out]
        n437 = property class="Enum (严格)"(reference=w769) -> ("Value"=w768:enum16{"总磷", "总氮"})  [unwired: 1 in, 2 out]
        n438 = property class="Enum (严格)"(reference=w770) -> ("Value"=w767:enum16{"水样测量", "零点核查", "跨度核查", "标样核查", "加标回收"})  [unwired: 1 in, 2 out]
        n439 = property class="Enum (严格)"(reference=w771) -> ("Value"=w766:enum16{"低量程", "高量程"})  [unwired: 1 in, 2 out]
        n440 = call "总磷总氮量程读取.vi"("量程"=w766, "测量模式"=w767, "测量参数"=w768) -> ("error out"=w762:errorcluster, "量程切换阈值"=w764:cluster{"阈值":dbl, "标液浓度":dbl})  [unwired: 7 in]
        n441 = property class="Clust (严格)"(reference=w765, "Value"=w764) -> ()  [unwired: 1 in, 2 out]
        n442 = case shown="错误" w762 {
          tunnel: ["读取成功" ("消息") "读取失败" ("消息")] -> w763
          frame No Error {
          }
          frame Error {
          }
        }
        n443 = One Button Dialog(message=w763) -> ()  [unwired: 1 in, 1 out]
      }
      event "量程切换阈值写入": Value Change {
        n444 = event-data() -> ()  [unwired: 1 in, 6 out]
        n445 = property class="Enum (严格)"(reference=w782) -> ("Value"=w779:enum16{"总磷", "总氮"})  [unwired: 1 in, 2 out]
        n446 = property class="Enum (严格)"(reference=w781) -> ("Value"=w778:enum16{"水样测量", "零点核查", "跨度核查", "标样核查", "加标回收"})  [unwired: 1 in, 2 out]
        n447 = property class="Enum (严格)"(reference=w780) -> ("Value"=w777:enum16{"低量程", "高量程"})  [unwired: 1 in, 2 out]
        n448 = call "总磷总氮量程写入.vi"("量程切换阈值"="量程切换阈值", "量程"=w777, "测量模式"=w778, "测量参数"=w779) -> ("error out"=w774:errorcluster)  [unwired: 7 in]
        n449 = case shown="无错误" w774 {
          tunnel: ["写入成功" ("消息") "写入失败" ("消息")] -> w775
          frame No Error {
          }
          frame Error {
          }
        }
        n450 = One Button Dialog(message=w775) -> ()  [unwired: 1 in, 1 out]
      }
      event "备用系数读取": Value Change {
        n451 = event-data() -> ()  [unwired: 1 in, 6 out]
        n452 = property class="Enum (严格)"(reference=w794) -> ("Value"=w793:enum16{"总磷", "总氮"})  [unwired: 1 in, 2 out]
        n453 = property class="Enum (严格)"(reference=w787) -> ("Value"=w786:enum16{"水样测量", "零点核查", "跨度核查", "标样核查", "加标回收"})  [unwired: 1 in, 2 out]
        n454 = property class="Enum (严格)"(reference=w788) -> ("Value"=w785:enum16{"低量程", "高量程"})  [unwired: 1 in, 2 out]
        n455 = call "总磷总氮备用系数读取.vi"("量程"=w785, "测量模式"=w786, "测量参数"=w793) -> ("error out"=w789:errorcluster, "备用系数"=w791:T2)  [unwired: 7 in]
        n456 = property class="Clust (严格)"(reference=w792, "Value"=w791) -> ()  [unwired: 1 in, 2 out]
        n457 = case shown="错误" w789 {
          tunnel: ["读取成功" ("消息") "读取失败" ("消息")] -> w790
          frame No Error {
          }
          frame Error {
          }
        }
        n458 = One Button Dialog(message=w790) -> ()  [unwired: 1 in, 1 out]
      }
      event "备用系数写入": Value Change {
        n459 = event-data() -> ()  [unwired: 1 in, 6 out]
        n460 = property class="Enum (严格)"(reference=w805) -> ("Value"=w804:enum16{"总磷", "总氮"})  [unwired: 1 in, 2 out]
        n461 = property class="Enum (严格)"(reference=w800) -> ("Value"=w798:enum16{"水样测量", "零点核查", "跨度核查", "标样核查", "加标回收"})  [unwired: 1 in, 2 out]
        n462 = property class="Enum (严格)"(reference=w799) -> ("Value"=w797:enum16{"低量程", "高量程"})  [unwired: 1 in, 2 out]
        n463 = call "总磷总氮备用系数写入.vi"("备用系数"="备用系数", "量程"=w797, "测量模式"=w798, "测量参数"=w804) -> ("error out"=w801:errorcluster)  [unwired: 7 in]
        n464 = case shown="无错误" w801 {
          tunnel: ["写入成功" ("消息") "写入失败" ("消息")] -> w802
          frame No Error {
          }
          frame Error {
          }
        }
        n465 = One Button Dialog(message=w802) -> ()  [unwired: 1 in, 1 out]
      }
    }
  }
